vi "STORE_INPUT.vi"(9 "CURRENT_YEAR_DATA":string, 10 "connection reference":T1, 11 "ECODE 2":string) -> ()   [LabVIEW 2015]
uses:
  <vilib>/addons/database/Connection.llb/Conn ObjectReference.ctl
  <vilib>/Utility/miscctls.llb/LVRowAndColumnUnsignedTypeDef.ctl
  Controls/STORE_INPUT_NO_CLUSTER.ctl
  Controls/STORE_INPUT_INFORMATION_Cluster.ctl
  Controls/ITEM_INFORMATION_CLUSTER.ctl
  Controls/Print_Data.ctl
  <vilib>/addons/database/Connection.llb/Conn Execute.vi
  <vilib>/addons/database/Recordset.llb/Rec Destroy - Connection.vi
  <vilib>/addons/database/_DB Variant To Data/Database Variant To Data.xnode
  <vilib>/addons/database/NI_Database_API.lvlib
  <vilib>/addons/database/Connection.llb/DB Tools Open Connec (String).vi
panel:
  in  "AUTO_PRINT":bool caption="AUTO"
  in  "PRINT button":bool
  in  "Lot Maker":string
  in  "Next Button":bool
  out "Find Array":i32[](array[numeric])
  in  "Location":string
  in  "Maker Code":string
  in  "Excle Path (F1)":path
  in  "BUTTON_EXIT":bool
  in  "BUTTON_INPUT":bool
  in  "BUTTON_ADD":bool
  in  "Search":string
  in  "Amount (F4)":dbl caption="(F4)"
  in  "Unit 2":string
  in  "Quantity":dbl
  in  "Lot Size":dbl
  in  "Unit":string
  in  "Item Code (F3)":string
  in  "Part No (F2)":string
  in  "Barcode (F1)":string
  in  "Offset":dbl
  in  "Length":dbl
  in  "Maker":string(combo)
  in  "Part Name":string(combo)
  in  "Product":string(combo)
  out "ECODE":string
  in  "Input Date":timestamp format="%<%d/%m/%Y>T"
  out "Input No.":string
  out "Table":string[][](table)
  # "INPUT"
  # "X"
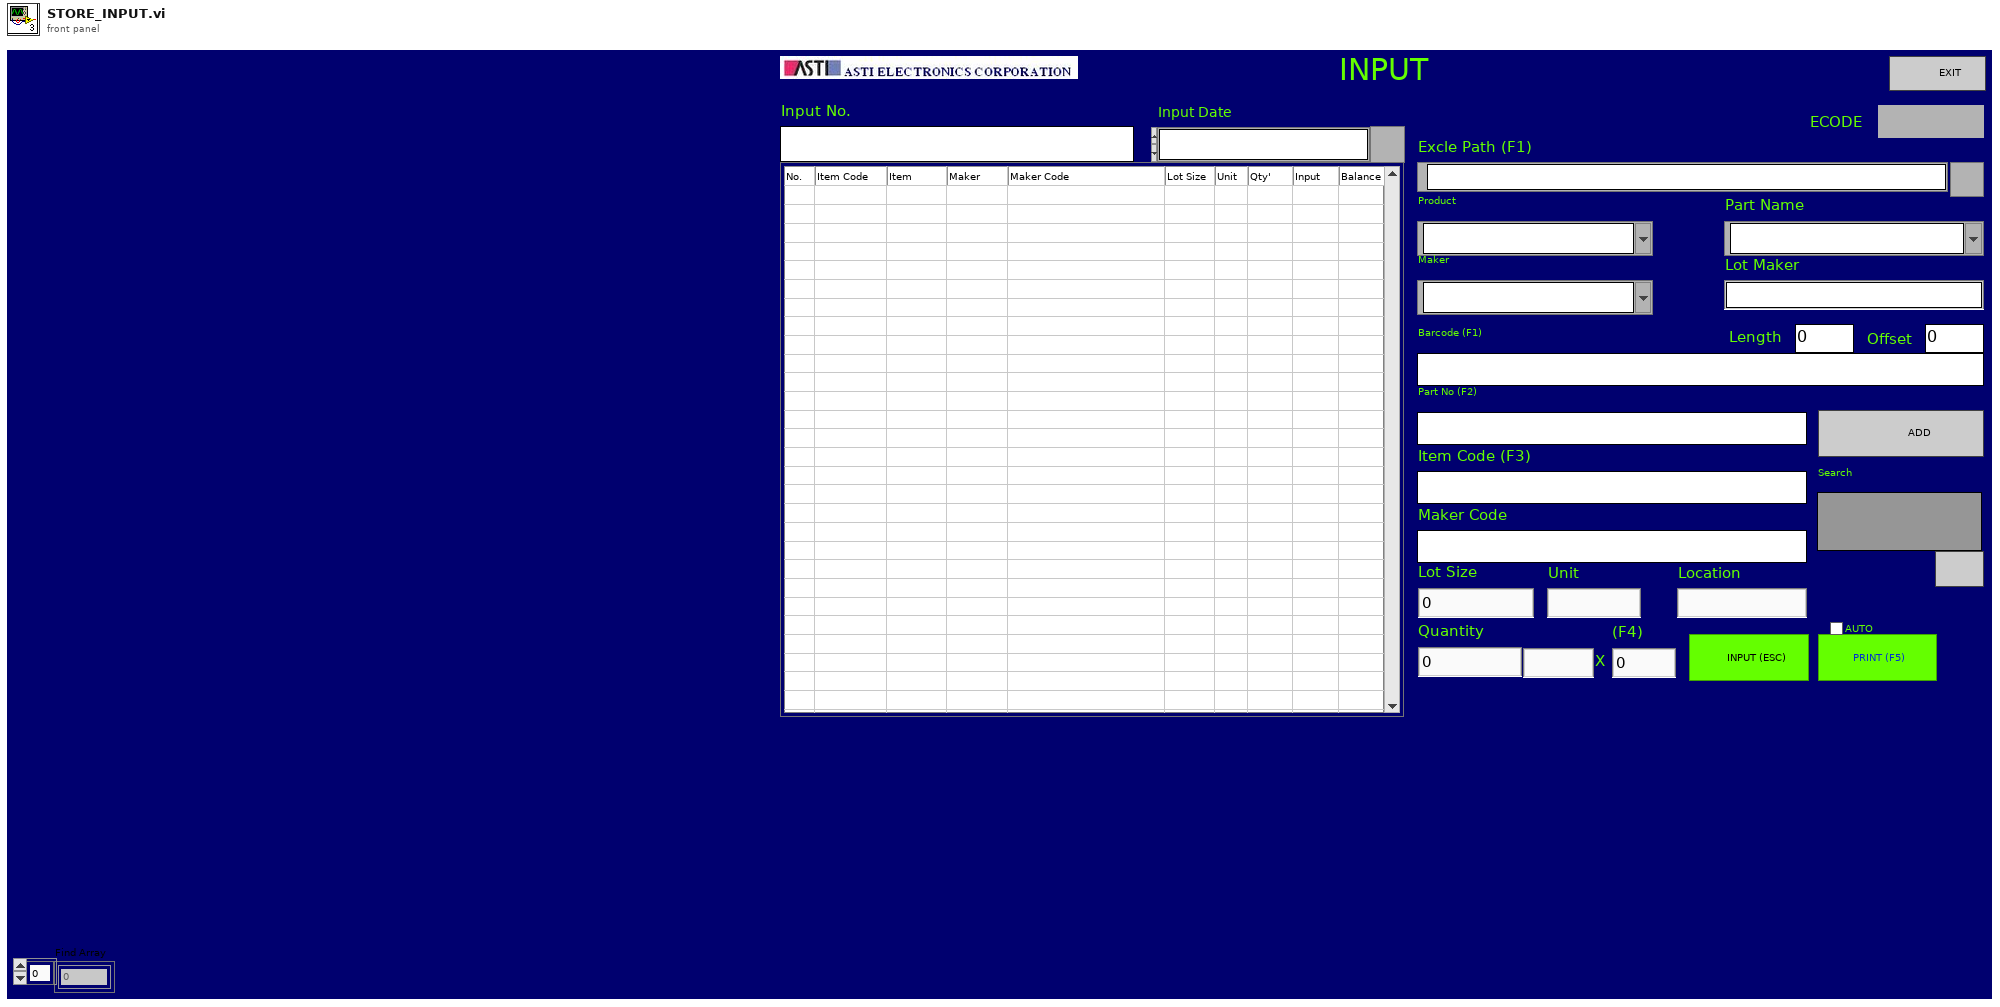
[diagram p1: front panel]
types:
  T1 = typedef "NI_Database_API.lvlib/Conn ObjectReference.ctl" = refnum<k1>
  T2 = typedef "LVRowAndColumnUnsignedTypeDef.ctl" = cluster{"Row":u32, "Column":u32}
  T3 = typedef "STORE_INPUT_NO_CLUSTER.ctl" = cluster{"NO":dbl, "ITEM_CODE":string, "ITEM":string, "MAKER":string, "MAKER_CODE":string, "LOT_SIZE":dbl, "UNIT":string, "QUANTITY":dbl, "INPUT":dbl, "BALANCE":dbl, "DESTINATION":string, "INVOICE_NO":string}
  T4 = cluster{"start (-1, -1)":cluster{"row":i32, "column":i32}, "end (-1, -1)":cluster{"row":i32, "column":i32}}
  T5 = typedef "STORE_INPUT_INFORMATION_Cluster.ctl" = cluster{"INPUT_NO":string, "INPUT_DATE":timestamp, "ECODE":string}
  T6 = typedef "ITEM_INFORMATION_CLUSTER.ctl" = cluster{"PRODUCT":string, "ITEM_CODE":string, "PART_NAME":string, "MAKER":string, "PART_NO":string, "LOT_SIZE":dbl, "UNIT":string, "LENGTH-OFFSET":string, "BARCODE":string, "PROCESS":string, "INVENTORY_LOCAL":string, "TARE":dbl, "SAMPLE":dbl}
  T7 = typedef "Print_Data.ctl" = cluster{"QR_code Text":string, "Lot Maker":string, "Item Code (F3)":string, "date/time string":string, "Invoice No.":string, "Maker":string, "Part No.(F2) ":string, "Location":string, "Product":string, "Qty":string, "ECODE":string}
  T8 = cluster{"ITEM_CODE":string, "INVOICE_NO":string, "INVOICE_DATE":timestamp, "LOT_MAKER":string, "QUANTITY":dbl, "INVOICE_ECODE":string, "INPUT_NO":string, "INPUT_DATE":timestamp, "INPUT_ECODE":string, "LINEBACK_NO":string, "LINEBACK_DATE":timestamp, "LINEBACK_ECODE":string, "OUTPUT_NO":string, "OUTPUT_DATE":timestamp, "OUTPUT_ECODE":string, "DESTINATION":string}
  T9 = cluster{"PRODUCT":string, "ITEM CODE":string, "PART NAME":string, "MAKER":string, "PART NO":string, "LOT SIZE":dbl, "UNIT":string, "LENGTH-OFFSET":string, "BARCODE":string, "PROCESS":string, "INVENTORY LOCAL":string, "TARE":dbl, "SAMPLE":dbl}
  T10 = typedef "NI_Database_API.lvlib/Rec ObjectReference.ctl" = refnum<k1>
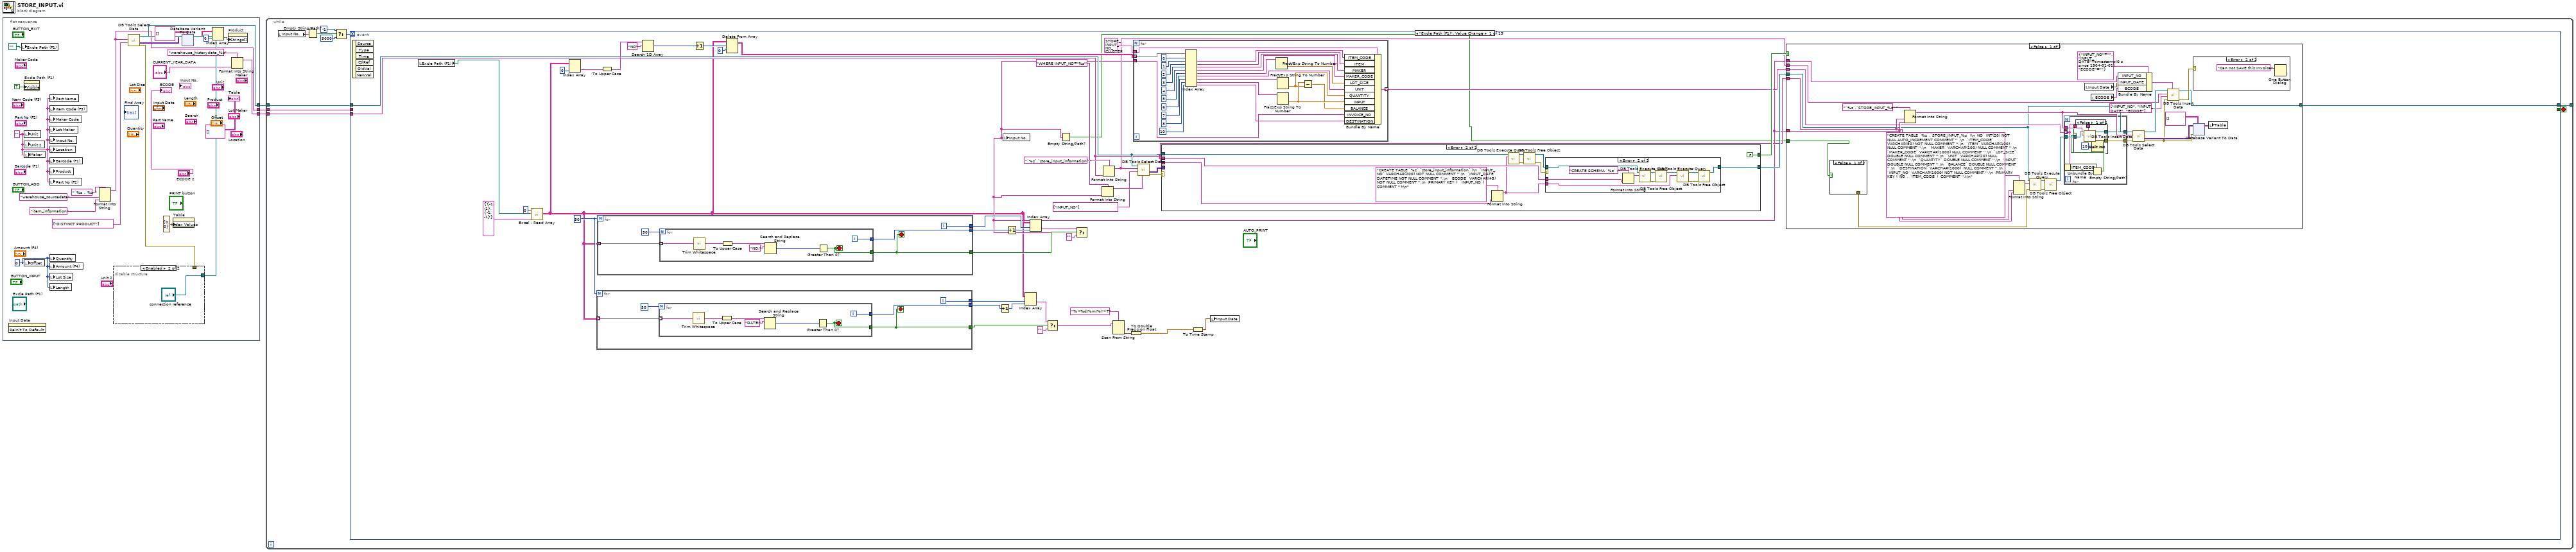
[diagram p0: block diagram]
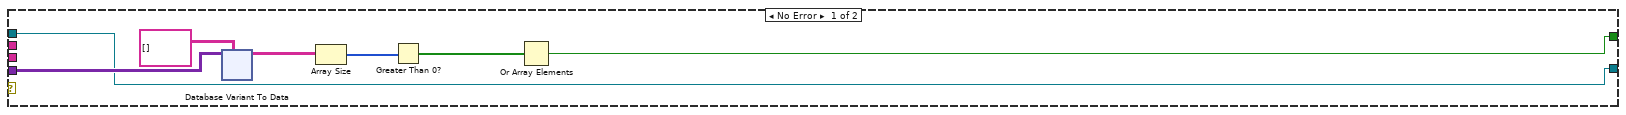
[diagram p2: hidden frame]
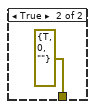
[diagram p4: hidden frame]
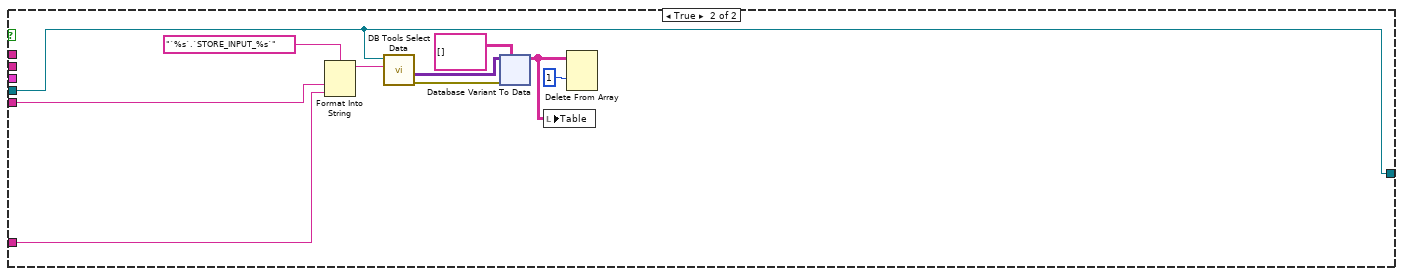
[diagram p7: hidden frame]
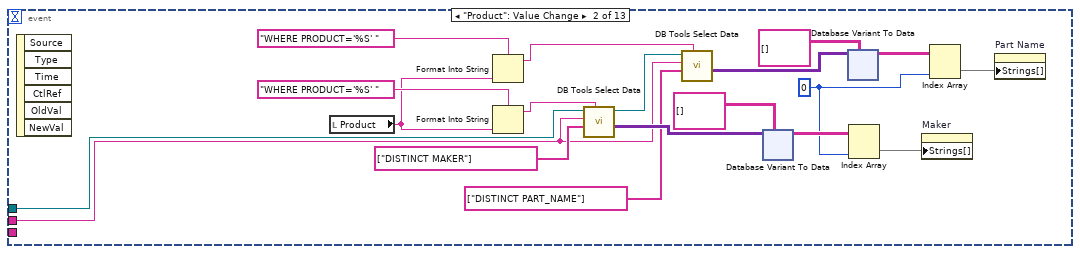
[diagram p8: hidden frame]
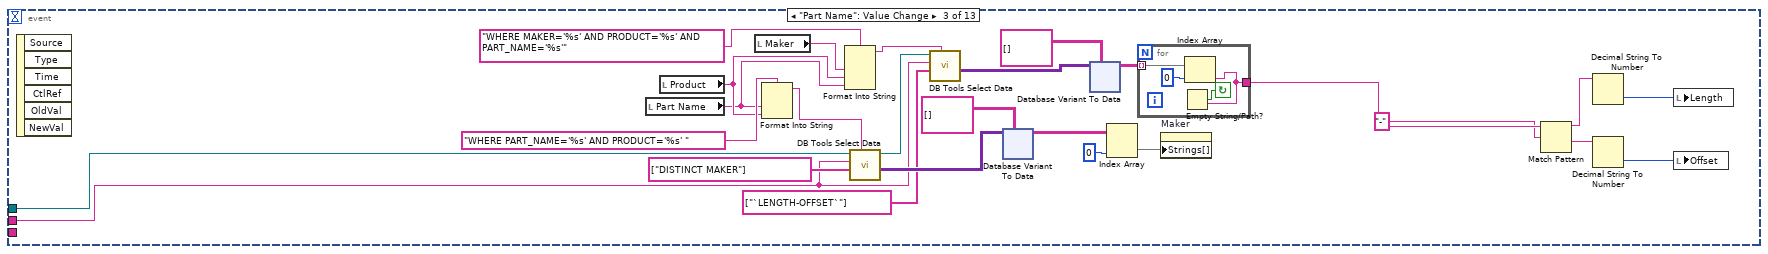
[diagram p9: hidden frame]
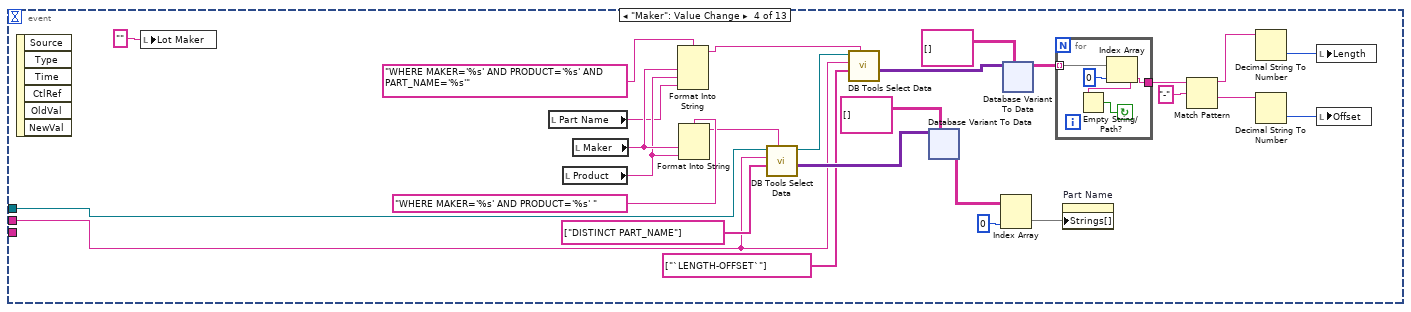
[diagram p10: hidden frame]
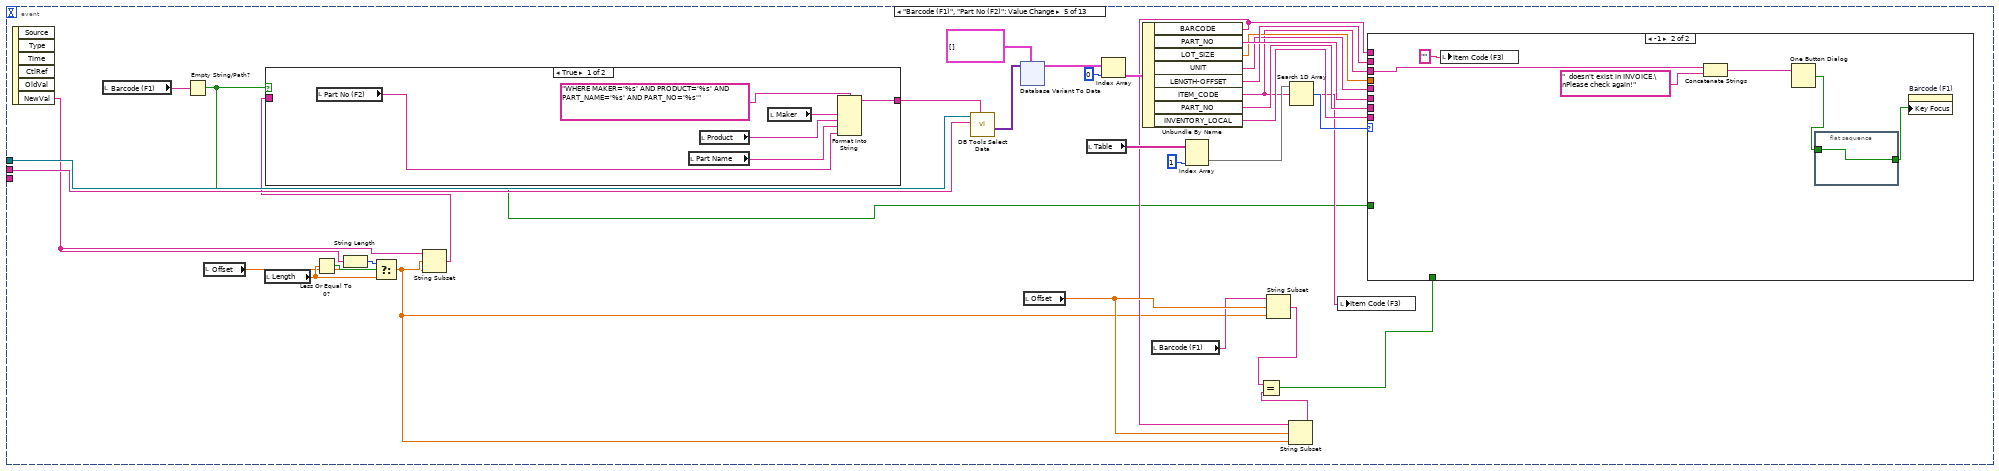
[diagram p11: hidden frame]
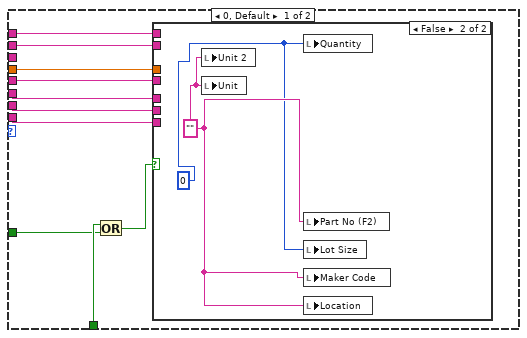
[diagram p12: hidden frame]
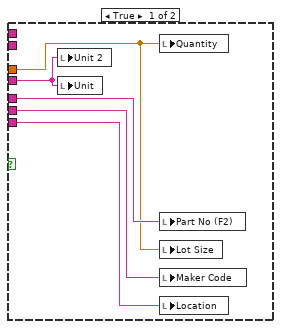
[diagram p13: hidden frame]
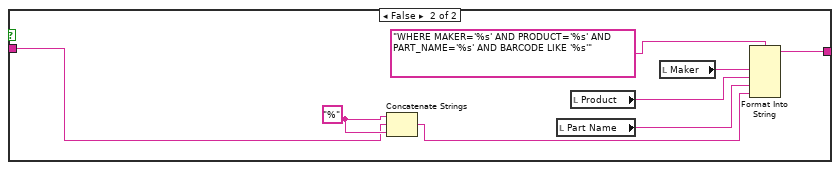
[diagram p14: hidden frame]
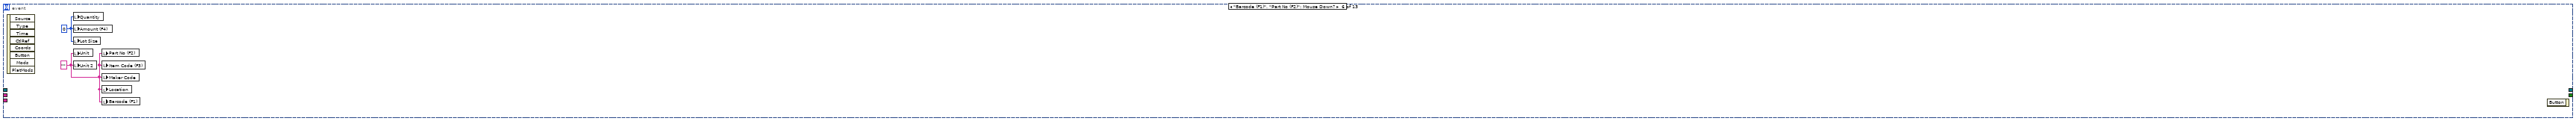
[diagram p15: hidden frame]
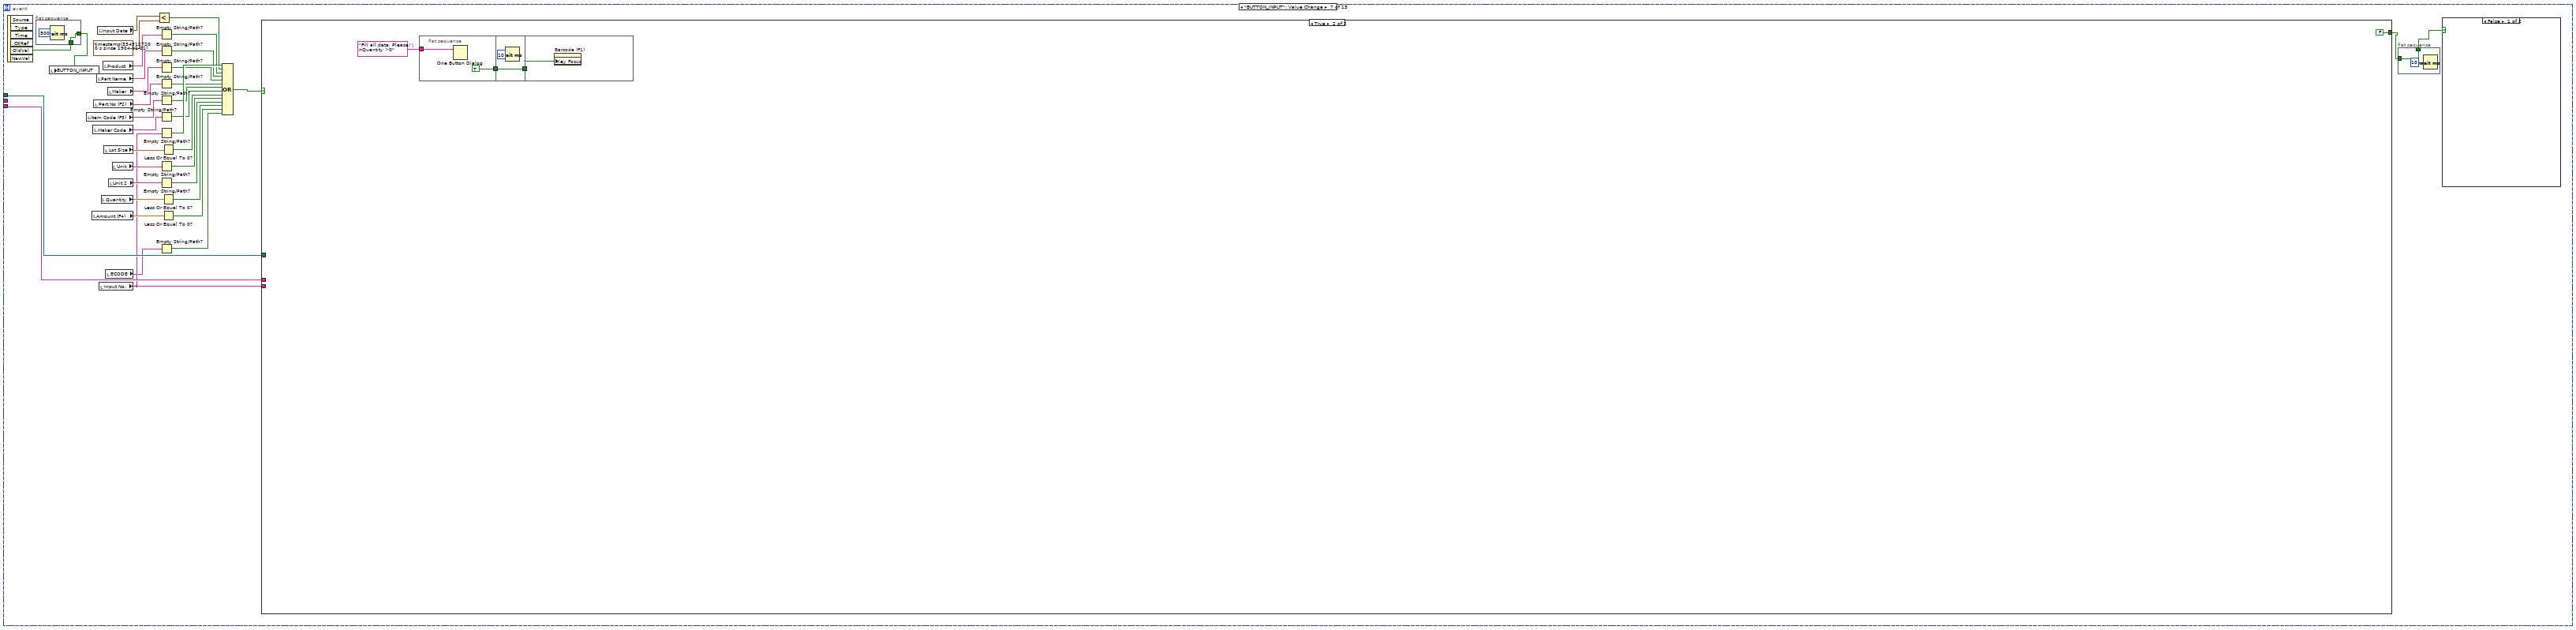
[diagram p16: hidden frame]
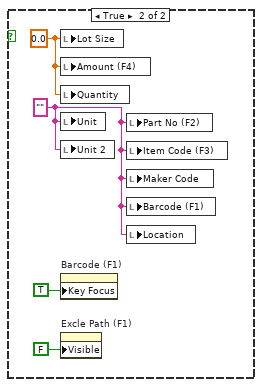
[diagram p17: hidden frame]
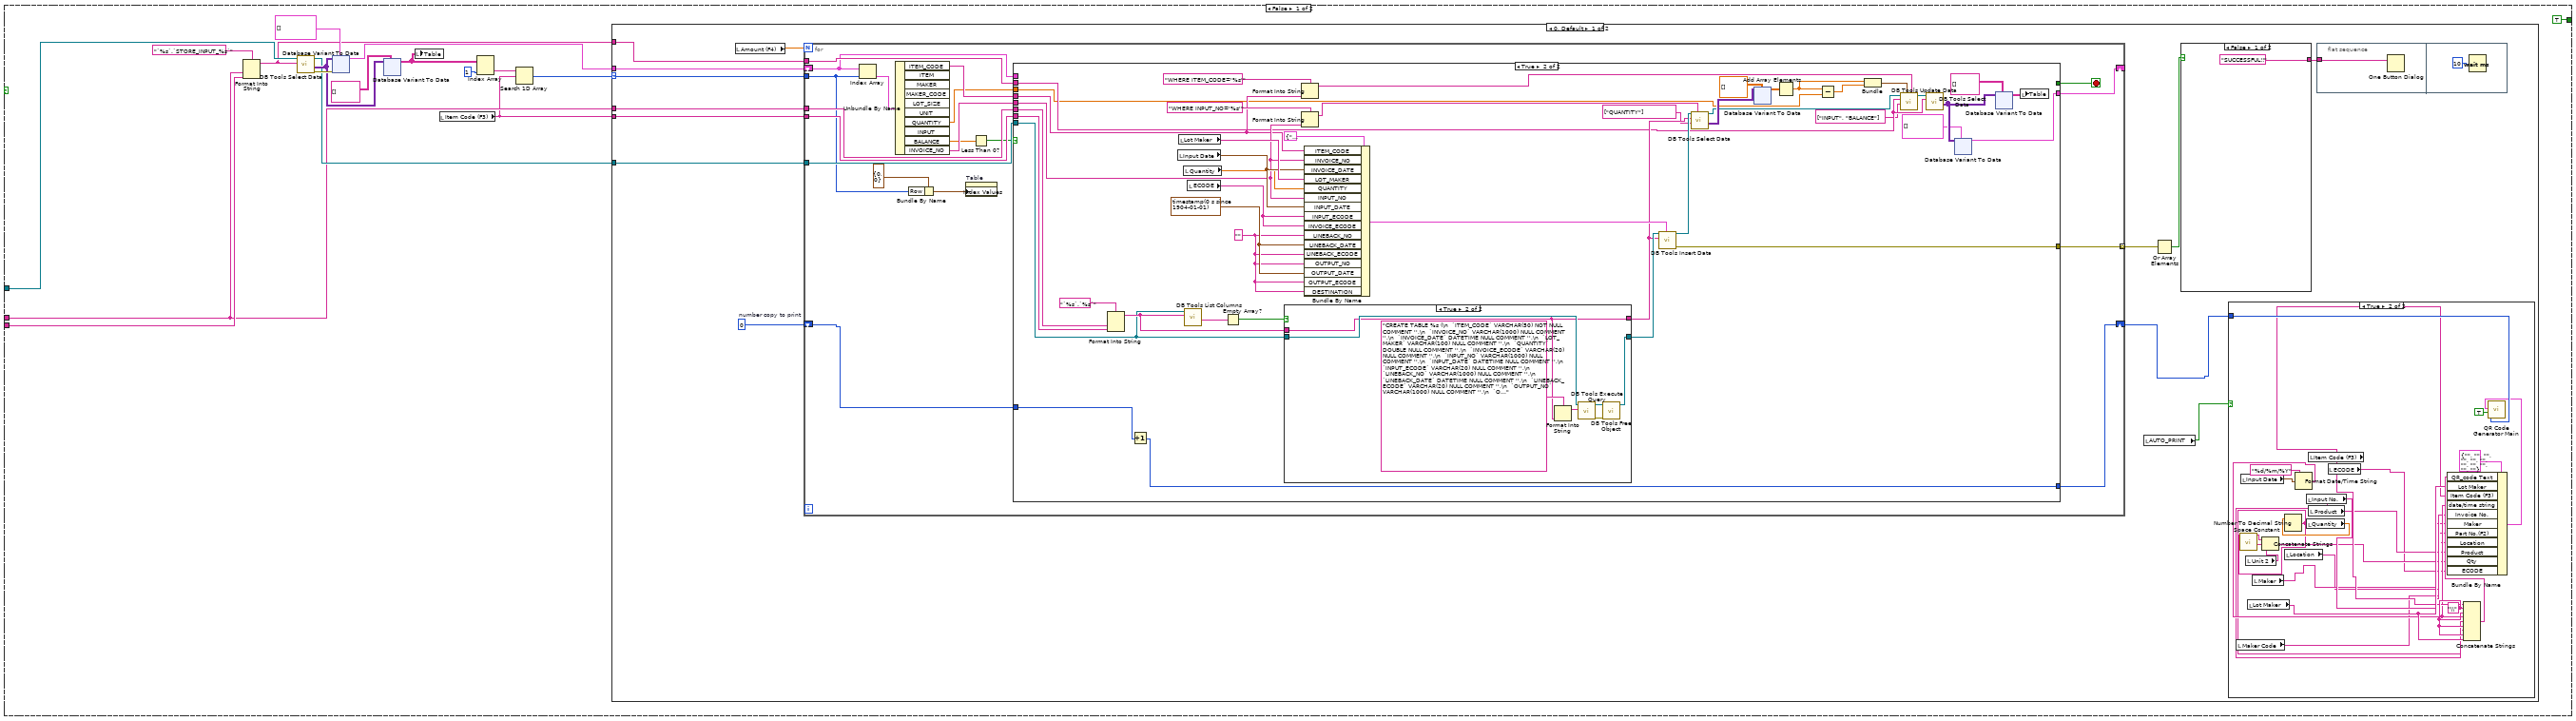
[diagram p18: hidden frame]
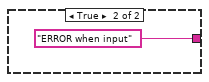
[diagram p20: hidden frame]
diagram:
  n1 = flat-sequence {
    tunnel: [w22] -> w3
    tunnel: [w16] -> w2
    tunnel: [w12] -> w1
    frame #0 {
      w10 = 0
      w8 = ""
      n2 = invoke on="Input Date" class="AbsTime (strict)" method="Reinit To Default"() -> ()  [unwired: 3 in, 3 out]
      n3 = local write "Excle Path (F1)"(path "" ("Excle Path")) -> ()
      n4 = property on="Excle Path (F1)" class="Path"("Visible"=TRUE) -> ()  [unwired: 2 in, 2 out]
      n5 = local write "Unit"(w8) -> ()
      n6 = local write "Unit 2"(w8) -> ()
      n7 = local write "Maker"(w8) -> ()
      n8 = local write "Offset"(w10) -> ()
      n9 = local write "Part Name"(w8) -> ()
      n10 = local write "Item Code (F3)"(w8) -> ()
      n11 = local write "Maker Code"(w8) -> ()
      n12 = local write "Lot Maker"(w8) -> ()
      n13 = local write "Input No."(w8) -> ()
      n14 = local write "Location"(w8) -> ()
      n15 = local write "Barcode (F1)"(w8) -> ()
      n16 = local write "Product"(w8) -> ()
      n17 = local write "Part No (F2)"(w8) -> ()
      n18 = local write "Quantity"(w10) -> ()
      n19 = local write "Amount (F4)"(w10) -> ()
      n20 = local write "Lot Size"(w10) -> ()
      n21 = local write "Length"(w10) -> ()
      n22 = Format Into String(format string="`%s`.`%s`" ("table"), "warehouse_sourcedata" ("table"), "item_information" ("table")) -> (resulting string=w16:string)  [unwired: 2 in, 1 out]
      n23 = disable-structure shown="Enabled" {
        disable-tunnel: [w28 "connection reference"] -> w24
        disable-tunnel: [w27 _] -> w23
        frame Disabled {
          n24 = call-poly <vilib>:"DB Tools Open Connection.vi"("password"="871994" ("userID"), "userID"="hoangbao2106", "connection information"="Database" ("userID")) -> ("error out"=w27:errorcluster, "connection reference"=w28:T1)  [unwired: 5 in]
        }
        frame Enabled {
        }
      }
      n25 = call <vilib>:"DB Tools Select Data.vi"("error in (no error)"=w23, "columns"=string[] ["DISTINCT PRODUCT"], "table"=w16, "connection reference"=w24) -> ("data"=w21:variant[][], "connection reference out"=w22:T1)  [unwired: 2 in, 1 out]
      n26 = property on="Table" class="Tbl (strict)"("Index Values"=T2 {"Row"=0, "Column"=0}) -> ()  [unwired: 2 in, 2 out]
      n27 = xnode "Database Variant To Data"("database variant"=w21, "type"=string[][] []) -> ("data"=w18:string[][])  [unwired: 1 in, 1 out]
      n28 = Index Array(array=w18, index (col)=0 ("index (row)")) -> (element=w17:string[])  [unwired: 1 in]
      n29 = property on="Product" class="CmbBox"("Strings[]"=w17) -> ()  [unwired: 2 in, 2 out]
      n30 = Format Into String(format string="warehouse_historydata_%s" ("table"), "CURRENT_YEAR_DATA") -> (resulting string=w12:string)  [unwired: 2 in, 1 out]
      "Table" <- string[][] [] ("Table")
      "ECODE" <- "ECODE 2"
    }
  }
  n31 = while {
    tunnel: w3 -> [w85]
    tunnel: w2 -> [w84]
    tunnel: w1 -> [w83]
    tunnel: [w82] -> _
    stop <- w86 stop-if-true
    n32 = local read "Input No."() -> (w81:string)
    n33 = Empty String/Path?(string/path=w81) -> (empty?=w80:bool)
    n34 = Select(t=-1, s=w80, f=5000) -> (s? t:f=w78:i32)
    n35 = event shown="[0] \"Excle Path (F1)\": Value Change" {
      selector: _ -> [_ _ _ _ _ _ _ _ _ _ _ _ _]
      dyn-events: _ -> [_ _ _ _ _ _ _ _ _ _ _ _ _]
      timeout: w78 -> [_ _ _ _ _ _ _ _ _ _ _ _ _]
      tunnel: [_ _ _ _ _ _ _ _ _ _ _ _ TRUE] -> w86
      tunnel: w85 -> [w110 w414 w525 w644 w775 _ w1239 _ w2362 w2395 _ _ _]
      tunnel: w84 -> [_ w401 w510 w640 w774 _ _ _ _ _ _ _ _]
      tunnel: w83 -> [w108 _ _ _ _ _ w1238 _ _ w2394 _ _ _]
      tunnel: [w103 _ _ _ _ _ _ _ _ _ _ _ _] -> w82
      event "Excle Path (F1)": Value Change {
        w100 = 50
        n36 = event-data() -> ()  [unwired: 1 in, 6 out]
        n37 = local read "Excle Path (F1)"() -> (w132:path)
        n38 = call "Excel - Read Array.vi"("Cluster"=T4 {"start (-1, -1)"={"row"=-1, "column"=-1}, "end (-1, -1)"={"row"=-1, "column"=-1}}, "Path"=w132, "worksheet index (0)"=0) -> ("Element 1"=w99:string[][])  [unwired: 5 in, 1 out]
        n39 = Index Array(array=w99, index (col)=0 ("disabled index (col)")) -> (element=w122:string[])  [unwired: 1 in]
        n40 = for {
          N: w100 -> [_]
          tunnel: w99 -> [w137] mode=indexing
          tunnel: [w136] -> w98
          tunnel: [w134] -> w97
          tunnel: [w133] -> w94
          i -> [w136]
          stop <- w133 stop-if-true
          n41 = for {
            N: 50 -> [_]
            tunnel: w137 -> [w143] mode=indexing
            tunnel: [w138] -> w133
            tunnel: [w144] -> w134
            i -> [w144]
            stop <- w138 stop-if-true
            n42 = call <vilib>:"Trim Whitespace.vi"("string"=w143) -> ("trimmed string"=w142:string)  [unwired: 1 in]
            n43 = To Upper Case(1:w142) -> (0:w141:string)
            n44 = Search and Replace String(input string=w141, search string="DATE:" ("y")) -> (number of replacements=w139:i32)  [unwired: 6 in, 3 out]
            n45 = Greater Than 0?(x=w139) -> (x > 0?=w138:bool)
          }
        }
        n46 = for {
          N: w100 -> [_]
          tunnel: w99 -> [w392] mode=indexing
          tunnel: [w391] -> w127
          tunnel: [w389] -> w129
          tunnel: [w388] -> w130
          i -> [w391]
          stop <- w388 stop-if-true
          n47 = for {
            N: 50 -> [_]
            tunnel: w392 -> [w398] mode=indexing
            tunnel: [w393] -> w388
            tunnel: [w399] -> w389
            i -> [w399]
            stop <- w393 stop-if-true
            n48 = call <vilib>:"Trim Whitespace.vi"("string"=w398) -> ("trimmed string"=w397:string)  [unwired: 1 in]
            n49 = To Upper Case(1:w397) -> (0:w396:string)
            n50 = Search and Replace String(input string=w396, search string="NO:" ("y")) -> (number of replacements=w394:i32)  [unwired: 6 in, 3 out]
            n51 = Greater Than 0?(x=w394) -> (x > 0?=w393:bool)
          }
        }
        n52 = To Upper Case(1:w122) -> (0:w121:string[])
        n53 = Search 1D Array(1D array=w121, element="NO") -> (index of element=w120:i32)  [unwired: 1 in]
        n54 = Increment(x=w120) -> (x+1=w119:i32)
        n55 = Delete From Array(array=w99, length=w119, index (row)=0) -> (array with subset deleted=w107:string[][])  [unwired: 1 in, 1 out]
        n56 = Increment(x=w97) -> (x+1=w96:i32)
        n57 = Increment(x=w129) -> (x+1=w128:i32)
        n58 = Index Array(array=w99, index (row)=w98, index (col)=w96) -> (element=w93:string)
        n59 = Index Array(array=w99, index (row)=w127, index (col)=w128) -> (element=w126:string)
        n60 = Select(t=w93, s=w94, f="") -> (s? t:f=w90:string)
        n61 = Select(t=w126, s=w130, f="") -> (s? t:f=w102:string)
        n62 = local write "Input No."(w102) -> ()
        n63 = Empty String/Path?(string/path=w102) -> (empty?=w101:bool)
        n64 = Format Into String(format string="WHERE INPUT_NO='%s'", w102) -> (resulting string=w115:string)  [unwired: 2 in, 1 out]
        n65 = Format Into String(format string="`%s`.`store_input_information` ", w108) -> (resulting string=w104:string)  [unwired: 2 in, 1 out]
        n66 = Scan From String(format string="%<%d/%m/%Y>T", input string=w90) -> (output 1=w91:timestamp)  [unwired: 3 in, 3 out]
        n67 = To Double Precision Float(number=w91) -> (double precision float=w89:dbl)
        n68 = for {
          tunnel: w107 -> [w170] mode=indexing
          tunnel: T3 {"NO"=0.0, "ITEM_CODE"="", "ITEM"="", "MAKER"="", "MAKER_CODE"="", "LOT_SIZE"=0.0, "UNIT"="", "QUANTITY"=0.0, "INPUT"=0.0, "BALANCE"=0.0, "DESTINATION"="", "INVOICE_NO"=""} -> [w171]
          tunnel: [w150] -> w105 mode=indexing
          tunnel: w102 -> [w149]
          n69 = Index Array(array=w170, index #1=0 ("index"), index #2=1 ("index"), index #3=2 ("index"), index #4=3 ("index"), index #5=4 ("index"), index #6=5 ("index"), index #7=6 ("index"), index #8=7 ("index"), index #9=8 ("index"), index #10=10 ("index")) -> (element #2=w159:string, element #3=w158:string, element #4=w157:string, element #5=w156:string, element #6=w155:string, element #7=w153:string, element #8=w152:string, element #9=w151:string, element #10=w145:string)  [unwired: 1 out]
          n70 = Fract/Exp String To Number(string=w155) -> (number=w154:dbl)  [unwired: 3 in, 1 out]
          n71 = Fract/Exp String To Number(string=w152) -> (number=w147:dbl)  [unwired: 3 in, 1 out]
          n72 = Fract/Exp String To Number(string=w151) -> (number=w148:dbl)  [unwired: 3 in, 1 out]
          n73 = Subtract(x=w148, y=w147) -> (x-y=w146:dbl)
          n74 = Bundle By Name(cluster=w171, "ITEM_CODE"=w159, "ITEM"=w158, "MAKER"=w157, "MAKER_CODE"=w156, "LOT_SIZE"=w154, "UNIT"=w153, "QUANTITY"=w147, "INPUT"=w148, "BALANCE"=w146, "INVOICE_NO"=w149, "DESTINATION"=w145) -> (w150:T3)
        }
        n75 = call <vilib>:"DB Tools Select Data.vi"("condition"=w115, "columns"=string[] ["INPUT_NO"], "table"=w104, "connection reference"=w110) -> ("error out"=w111:errorcluster, "data"=w114:variant[][])  [unwired: 2 in, 1 out]
        n76 = case shown="Error" w111 {
          tunnel: w114 -> [w178 _]
          tunnel: [w173 FALSE] -> w112
          tunnel: w110 -> [w172 w230]
          tunnel: [w172 w226] -> w109
          tunnel: w108 -> [_ w228]
          tunnel: w108 -> [_ w224]
          frame No Error {
            n77 = xnode "Database Variant To Data"("database variant"=w178, "type"=string[][] []) -> ("data"=w176:string[][])  [unwired: 1 in, 1 out]
            n78 = Array Size(array=w176) -> (size(s)=w175:i32[])
            n79 = Greater Than 0?(x=w175) -> (x > 0?=w174:bool[])
            n80 = Or Array Elements(Boolean array=w174) -> (logical OR=w173:bool)
          }
          frame Error {
            n81 = Format Into String(format string="CREATE TABLE `%s`.`store_input_information` (\n  `INPUT_NO` VARCHAR(200) NOT NULL COMMENT '',\n  `INPUT_DATE` DATETIME NOT NULL COMMENT '',\n  `ECODE` VARCHAR(45) NOT NULL COMMENT '',\n  PRIMARY KEY (  `INPUT_NO`)  COMMENT '');\n", w224) -> (resulting string=w223:string)  [unwired: 2 in, 1 out]
            n82 = call-poly <vilib>:"DB Tools Execute Query.vi"("SQL query"=w223, "connection reference"=w230) -> ("error out"=w232:errorcluster, "recordset reference"=w233:T10)  [unwired: 6 in]
            n83 = call-poly <vilib>:"DB Tools Free Object.vi"("error in (no error)"=w232, "recordset reference"=w233) -> ("error out"=w229:errorcluster, "connection reference"=w227:T1)  [unwired: 8 in]
            n84 = case shown="Error" w229 {
              tunnel: w227 -> [w234 w245]
              tunnel: w228 -> [_ w243]
              tunnel: w223 -> [_ w237]
              tunnel: [w234 w236] -> w226
              frame No Error {
              }
              frame Error {
                n85 = Format Into String(format string="CREATE SCHEMA `%s` ;" ("SQL query"), w243) -> (resulting string=w235:string)  [unwired: 2 in, 1 out]
                n86 = call-poly <vilib>:"DB Tools Execute Query.vi"("SQL query"=w235, "connection reference"=w245) -> ("error out"=w241:errorcluster, "recordset reference"=w242:T10)  [unwired: 6 in]
                n87 = call-poly <vilib>:"DB Tools Free Object.vi"("error in (no error)"=w241, "recordset reference"=w242) -> ("connection reference"=w238:T1)  [unwired: 8 in, 1 out]
                n88 = call-poly <vilib>:"DB Tools Execute Query.vi"("SQL query"=w237, "connection reference"=w238) -> ("error out"=w240:errorcluster, "recordset reference"=w239:T10)  [unwired: 6 in]
                n89 = call-poly <vilib>:"DB Tools Free Object.vi"("error in (no error)"=w240, "recordset reference"=w239) -> ("connection reference"=w236:T1)  [unwired: 8 in, 1 out]
              }
            }
          }
        }
        n90 = To Time Stamp(1:w89) -> (0:w88:timestamp)
        n91 = local write "Input Date"(w88) -> ()
        n92 = case shown="False" w112 {
          tunnel: w109 -> [w246 w343]
          tunnel: w108 -> [w269 w337]
          tunnel: w102 -> [w268 w338]
          tunnel: [w255 w343] -> w103
          tunnel: w105 -> [w267 _]
          tunnel: w104 -> [w258 _]
          tunnel: w102 -> [w254 _]
          tunnel: w101 -> [w248 _]
          frame False {
            n93 = case shown="False" w248 {
              tunnel: [_ errorcluster {"status"=TRUE, "code"=0, "source"=""} ("error constant")] -> w247
              frame False {
              }
              frame True {
              }
            }
            n94 = Format Into String(format string="`%s`.`STORE_INPUT_%s` " ("SQL query"), w269, w268) -> (resulting string=w262:string)  [unwired: 2 in, 1 out]
            n95 = Format Into String(format string="CREATE TABLE `%s`.`STORE_INPUT_%s` (\n`NO` INT(20) NOT NULL AUTO_INCREMENT COMMENT '' ,\n  `ITEM_CODE` VARCHAR(50) NOT NULL COMMENT '',\n  `ITEM` VARCHAR(100) NULL COMMENT '',\n  `MAKER` VARCHAR(100) NULL COMMENT '',\n  `MAKER_CODE` VARCHAR(1000) NULL COMMENT '',\n  `LOT_SIZE` DOUBLE NULL COMMENT '',\n  `UNIT` VARCHAR(20) NULL COMMENT '',\n  `QUANTITY` DOUBLE NULL COMMENT '',\n  `INPUT` DOUBLE NULL COMMENT '',\n  `BALANCE` DOUBLE NULL COMMENT '',\n  `DESTINATION` VARCHAR(1000)  NULL COMMENT '',\n  `INPUT_NO` VARCHAR(1000) NOT NULL COMMENT '',\n  PRIMARY KEY (`NO`, `ITEM_CODE`)  COMMENT '');\n" ("SQL query"), w269, w268) -> (resulting string=w261:string)  [unwired: 2 in, 1 out]
            n96 = call-poly <vilib>:"DB Tools Execute Query.vi"("error in (no error)"=w247, "SQL query"=w261, "connection reference"=w246) -> ("error out"=w271:errorcluster, "recordset reference"=w272:T10)  [unwired: 5 in]
            n97 = call-poly <vilib>:"DB Tools Free Object.vi"("error in (no error)"=w271, "recordset reference"=w272) -> ("connection reference"=w263:T1)  [unwired: 8 in, 1 out]
            n98 = for {
              tunnel: w263 -> [w326]
              tunnel: w262 -> [w325]
              tunnel: w267 -> [w322] mode=indexing
              tunnel: [w324] -> _
              tunnel: [w323] -> w260
              n99 = Unbundle By Name(w322) -> ("ITEM_CODE"=w321:string)
              n100 = Empty String/Path?(string/path=w321) -> (empty?=w320:bool)
              n101 = case shown="False" w320 {
                tunnel: w326 -> [w332 w333]
                tunnel: w325 -> [w331 _]
                tunnel: w322 -> [w330 _]
                tunnel: [w329 w333] -> w324
                tunnel: [w328 _] -> w323
                frame False {
                  n102 = call <vilib>:"DB Tools Insert Data.vi"("data"=w330, "table"=w331, "connection reference"=w332) -> ("error out"=w328:errorcluster, "connection reference out"=w329:T1)  [unwired: 7 in]
                  n103 = Wait (ms)(milliseconds to wait=u32 10) -> ()  [unwired: 1 out]
                }
                frame True {
                }
              }
            }
            n104 = local read "Input Date"() -> (w253:timestamp)
            n105 = local read "ECODE"() -> (w252:string)
            n106 = Bundle By Name(cluster=T5 {"INPUT_NO"="", "INPUT_DATE"=timestamp(0 s since 1904-01-01), "ECODE"=""} ("INVOICE_INFORMATION_Cluster"), "INPUT_NO"=w254, "INPUT_DATE"=w253, "ECODE"=w252) -> (w251:T5)
            n107 = call <vilib>:"DB Tools Select Data.vi"("error in (no error)"=w260, "table"=w262, "connection reference"=w246) -> ("error out"=w257:errorcluster, "data"=w266:variant[][], "connection reference out"=w259:T1)  [unwired: 3 in]
            n108 = call <vilib>:"DB Tools Insert Data.vi"("data"=w251, "error in (no error)"=w257, "columns"=string[] ["INPUT_NO", "INPUT_DATE", "ECODE"], "table"=w258, "connection reference"=w259) -> ("error out"=w256:errorcluster, "connection reference out"=w255:T1)  [unwired: 5 in]
            n109 = case shown="Error" w256 {
              frame No Error {
              }
              frame Error {
                n110 = One Button Dialog(message="Can not SAVE this Invoice") -> ()  [unwired: 1 in, 1 out]
              }
            }
            n111 = xnode "Database Variant To Data"("database variant"=w266, "error in (no error)"=w257, "type"=string[][] []) -> ("data"=w264:string[][])  [unwired: 1 out]
            n112 = local write "Table"(w264) -> ()
          }
          frame True {
            n113 = Format Into String(format string="`%s`.`STORE_INPUT_%s`", w337, w338) -> (resulting string=w336:string)  [unwired: 2 in, 1 out]
            n114 = call <vilib>:"DB Tools Select Data.vi"("table"=w336, "connection reference"=w343) -> ("error out"=w340:errorcluster, "data"=w342:variant[][])  [unwired: 4 in, 1 out]
            n115 = xnode "Database Variant To Data"("database variant"=w342, "error in (no error)"=w340, "type"=string[][] []) -> ("data"=w335:string[][])  [unwired: 1 out]
            n116 = local write "Table"(w335) -> ()
            n117 = Delete From Array(array=w335, index (row)=1) -> ()  [unwired: 2 in, 2 out]
          }
        }
      }
      event "Product": Value Change {
        w400 = 0 ("index (row)")
        n118 = event-data() -> ()  [unwired: 1 in, 6 out]
        n119 = local read "Product"() -> (w405:string)
        n120 = Format Into String(format string="WHERE PRODUCT='%S' " ("condition"), w405) -> (resulting string=w411:string)  [unwired: 2 in, 1 out]
        n121 = Format Into String(format string="WHERE PRODUCT='%S' " ("condition"), w405) -> (resulting string=w412:string)  [unwired: 2 in, 1 out]
        n122 = call <vilib>:"DB Tools Select Data.vi"("condition"=w412, "columns"=string[] ["DISTINCT MAKER"], "table"=w401, "connection reference"=w414) -> ("data"=w415:variant[][], "connection reference out"=w404:T1)  [unwired: 2 in, 1 out]
        n123 = call <vilib>:"DB Tools Select Data.vi"("condition"=w411, "columns"=string[] ["DISTINCT PART_NAME"], "table"=w401, "connection reference"=w404) -> ("data"=w409:variant[][])  [unwired: 2 in, 2 out]
        n124 = xnode "Database Variant To Data"("database variant"=w415, "type"=string[][] []) -> ("data"=w418:string[][])  [unwired: 1 in, 1 out]
        n125 = xnode "Database Variant To Data"("database variant"=w409, "type"=string[][] []) -> ("data"=w406:string[][])  [unwired: 1 in, 1 out]
        n126 = Index Array(array=w418, index (col)=w400) -> (element=w402:string[])  [unwired: 1 in]
        n127 = property on="Maker" class="CmbBox"("Strings[]"=w402) -> ()  [unwired: 2 in, 2 out]
        n128 = Index Array(array=w406, index (col)=w400) -> (element=w403:string[])  [unwired: 1 in]
        n129 = property on="Part Name" class="CmbBox"("Strings[]"=w403) -> ()  [unwired: 2 in, 2 out]
      }
      event "Part Name": Value Change {
        n130 = event-data() -> ()  [unwired: 1 in, 6 out]
        n131 = local read "Part Name"() -> (w507:string)
        n132 = local read "Product"() -> (w508:string)
        n133 = local read "Maker"() -> (w509:string)
        n134 = Format Into String(format string="WHERE PART_NAME='%s' AND PRODUCT='%s' " ("condition"), w507, w508) -> (resulting string=w527:string)  [unwired: 2 in, 1 out]
        n135 = Format Into String(format string="WHERE MAKER='%s' AND PRODUCT='%s' AND PART_NAME='%s'" ("condition"), w509, w508, w507) -> (resulting string=w520:string)  [unwired: 2 in, 1 out]
        n136 = call <vilib>:"DB Tools Select Data.vi"("condition"=w527, "columns"=string[] ["DISTINCT MAKER"], "table"=w510, "connection reference"=w525) -> ("data"=w529:variant[][], "connection reference out"=w511:T1)  [unwired: 2 in, 1 out]
        n137 = call <vilib>:"DB Tools Select Data.vi"("condition"=w520, "columns"=string[] ["`LENGTH-OFFSET`"], "table"=w510, "connection reference"=w511) -> ("data"=w523:variant[][])  [unwired: 2 in, 2 out]
        n138 = xnode "Database Variant To Data"("database variant"=w529, "type"=string[][] []) -> ("data"=w532:string[][])  [unwired: 1 in, 1 out]
        n139 = xnode "Database Variant To Data"("database variant"=w523, "type"=string[][] []) -> ("data"=w518:string[][])  [unwired: 1 in, 1 out]
        n140 = Index Array(array=w532, index (col)=0 ("index (row)")) -> (element=w524:string[])  [unwired: 1 in]
        n141 = for {
          tunnel: w518 -> [w536] mode=indexing
          tunnel: [w534] -> w517
          stop <- w533 continue-if-true
          n142 = Index Array(array=w536, index=0 ("index (row)")) -> (element=w534:string)
          n143 = Empty String/Path?(string/path=w534) -> (empty?=w533:bool)
        }
        n144 = property on="Maker" class="CmbBox"("Strings[]"=w524) -> ()  [unwired: 2 in, 2 out]
        n145 = Match Pattern(string=w517, regular expression="-") -> (before substring=w515:string, after substring=w514:string)  [unwired: 1 in, 2 out]
        n146 = Decimal String To Number(string=w515) -> (number=w512:i32)  [unwired: 2 in, 1 out]
        n147 = Decimal String To Number(string=w514) -> (number=w513:i32)  [unwired: 2 in, 1 out]
        n148 = local write "Length"(w512) -> ()
        n149 = local write "Offset"(w513) -> ()
      }
      event "Maker": Value Change {
        n150 = event-data() -> ()  [unwired: 1 in, 6 out]
        n151 = local write "Lot Maker"("" ("Lot Maker")) -> ()
        n152 = local read "Part Name"() -> (w635:string)
        n153 = local read "Product"() -> (w636:string)
        n154 = local read "Maker"() -> (w637:string)
        n155 = Format Into String(format string="WHERE MAKER='%s' AND PRODUCT='%s' AND PART_NAME='%s'" ("condition"), w637, w636, w635) -> (resulting string=w634:string)  [unwired: 2 in, 1 out]
        n156 = Format Into String(format string="WHERE MAKER='%s' AND PRODUCT='%s' " ("condition"), w637, w636) -> (resulting string=w646:string)  [unwired: 2 in, 1 out]
        n157 = call <vilib>:"DB Tools Select Data.vi"("condition"=w646, "columns"=string[] ["DISTINCT PART_NAME"], "table"=w640, "connection reference"=w644) -> ("data"=w648:variant[][], "connection reference out"=w641:T1)  [unwired: 2 in, 1 out]
        n158 = call <vilib>:"DB Tools Select Data.vi"("condition"=w634, "columns"=string[] ["`LENGTH-OFFSET`"], "table"=w640, "connection reference"=w641) -> ("data"=w642:variant[][])  [unwired: 2 in, 2 out]
        n159 = xnode "Database Variant To Data"("database variant"=w648, "type"=string[][] []) -> ("data"=w651:string[][])  [unwired: 1 in, 1 out]
        n160 = Index Array(array=w651, index (col)=0 ("index (row)")) -> (element=w643:string[])  [unwired: 1 in]
        n161 = xnode "Database Variant To Data"("database variant"=w642, "type"=string[][] []) -> ("data"=w632:string[][])  [unwired: 1 in, 1 out]
        n162 = for {
          tunnel: w632 -> [w655] mode=indexing
          tunnel: [w653] -> w631
          stop <- w652 continue-if-true
          n163 = Index Array(array=w655, index=0 ("index (row)")) -> (element=w653:string)
          n164 = Empty String/Path?(string/path=w653) -> (empty?=w652:bool)
        }
        n165 = property on="Part Name" class="CmbBox"("Strings[]"=w643) -> ()  [unwired: 2 in, 2 out]
        n166 = Match Pattern(string=w631, regular expression="-") -> (before substring=w629:string, after substring=w628:string)  [unwired: 1 in, 2 out]
        n167 = Decimal String To Number(string=w629) -> (number=w626:i32)  [unwired: 2 in, 1 out]
        n168 = Decimal String To Number(string=w628) -> (number=w627:i32)  [unwired: 2 in, 1 out]
        n169 = local write "Length"(w626) -> ()
        n170 = local write "Offset"(w627) -> ()
      }
      event "Barcode (F1)", "Part No (F2)": Value Change {
        n171 = event-data() -> ("NewVal"=w755:string)  [unwired: 1 in, 5 out]
        n172 = local read "Barcode (F1)"() -> (w763:string)
        n173 = Empty String/Path?(string/path=w763) -> (empty?=w744:bool)
        n174 = local read "Offset"() -> (w753:dbl)
        n175 = local read "Length"() -> (w754:dbl)
        n176 = Less Or Equal To 0?(x=w754) -> (x <= 0?=w757:bool)
        n177 = String Length(string=w755) -> (length=w756:i32)
        n178 = Select(t=w756, s=w757, f=w754) -> (s? t:f=w745:dbl)
        n179 = String Subset(string=w755, offset (0)=w753, length (rest)=w745) -> (substring=w752:string)
        n180 = case shown="True" w744 {
          tunnel: [w805 w813] -> w776
          tunnel: w752 -> [_ w809]
          frame True {
            n181 = local read "Part No (F2)"() -> (w802:string)
            n182 = local read "Part Name"() -> (w806:string)
            n183 = local read "Product"() -> (w803:string)
            n184 = local read "Maker"() -> (w804:string)
            n185 = Format Into String(format string="WHERE MAKER='%s' AND PRODUCT='%s' AND PART_NAME='%s' AND PART_NO='%s'" ("condition"), w804, w803, w806, w802) -> (resulting string=w805:string)  [unwired: 2 in, 1 out]
          }
          frame False {
            w810 = "%"
            n186 = Concatenate Strings(w810, w809, w810) -> (w808:string)
            n187 = local read "Part Name"() -> (w814:string)
            n188 = local read "Product"() -> (w811:string)
            n189 = local read "Maker"() -> (w812:string)
            n190 = Format Into String(format string="WHERE MAKER='%s' AND PRODUCT='%s' AND PART_NAME='%s' AND BARCODE LIKE '%s'" ("condition"), w812, w811, w814, w808) -> (resulting string=w813:string)  [unwired: 2 in, 1 out]
          }
        }
        n191 = call <vilib>:"DB Tools Select Data.vi"("condition"=w776, "table"=w774, "connection reference"=w775) -> ("data"=w777:variant[][])  [unwired: 3 in, 2 out]
        n192 = xnode "Database Variant To Data"("database variant"=w777, "type"=T6[] []) -> ("data"=w772:T6[])  [unwired: 1 in, 1 out]
        n193 = local read "Offset"() -> (w749:dbl)
        n194 = local read "Table"() -> (w762:string[][])
        n195 = Index Array(array=w772, index=0) -> (element=w770:T6)
        n196 = Unbundle By Name(w770) -> ("BARCODE"=w748:string, "PART_NO"=w769:string, "LOT_SIZE"=w767:dbl, "UNIT"=w766:string, "LENGTH-OFFSET"=w768:string, "ITEM_CODE"=w758:string, "PART_NO"=w765:string, "INVENTORY_LOCAL"=w764:string)
        n197 = local read "Barcode (F1)"() -> (w747:string)
        n198 = Index Array(array=w762, index (col)=1 ("disabled index (col)")) -> (element=w760:string[])  [unwired: 1 in]
        n199 = String Subset(string=w747, offset (0)=w749, length (rest)=w745) -> (substring=w750:string)
        n200 = String Subset(string=w748, offset (0)=w749, length (rest)=w745) -> (substring=w751:string)
        n201 = Equal?(x=w750, y=w751) -> (x = y?=w746:bool)
        n202 = Search 1D Array(1D array=w760, element=w758) -> (index of element=w759:i32)  [unwired: 1 in]
        n203 = local write "Item Code (F3)"(w758) -> ()
        n204 = case shown="-1" w759 {
          tunnel: w769 -> [w787 _]
          tunnel: w768 -> [w786 _]
          tunnel: w767 -> [w785 _]
          tunnel: w766 -> [w784 _]
          tunnel: w765 -> [w783 _]
          tunnel: w764 -> [w782 _]
          tunnel: w748 -> [w781 _]
          tunnel: w758 -> [_ w798]
          tunnel: w746 -> [w779 _]
          tunnel: w744 -> [w778 _]
          frame 0, Default {
            n205 = Or(x=w779, y=w778) -> (x .or. y?=w780:bool)
            n206 = case shown="False" w780 {
              tunnel: w787 -> [w792 _]
              tunnel: w786 -> [_ _]
              tunnel: w785 -> [w791 _]
              tunnel: w784 -> [w790 _]
              tunnel: w783 -> [w789 _]
              tunnel: w782 -> [w788 _]
              tunnel: w781 -> [_ _]
              frame True {
                n207 = local write "Unit 2"(w790) -> ()
                n208 = local write "Unit"(w790) -> ()
                n209 = local write "Quantity"(w791) -> ()
                n210 = local write "Part No (F2)"(w792) -> ()
                n211 = local write "Lot Size"(w791) -> ()
                n212 = local write "Maker Code"(w789) -> ()
                n213 = local write "Location"(w788) -> ()
              }
              frame False {
                w793 = 0
                w794 = ""
                n214 = local write "Unit 2"(w794) -> ()
                n215 = local write "Unit"(w794) -> ()
                n216 = local write "Quantity"(w793) -> ()
                n217 = local write "Part No (F2)"(w794) -> ()
                n218 = local write "Lot Size"(w793) -> ()
                n219 = local write "Maker Code"(w794) -> ()
                n220 = local write "Location"(w794) -> ()
              }
            }
          }
          frame -1 {
            n221 = local write "Item Code (F3)"("" ("Item Code")) -> ()
            n222 = Concatenate Strings(w798, "  doesn't exist in INVOICE.\nPlease check again!" ("message")) -> (w797:string)
            n223 = One Button Dialog(message=w797) -> (true=w796:bool)  [unwired: 1 in]
            n224 = flat-sequence {
              tunnel: [w801] -> w795
              tunnel: w796 -> [w801]
              frame #0 {
              }
            }
            n225 = property on="Barcode (F1)" class="Str"("Key Focus"=w795) -> ()  [unwired: 2 in, 2 out]
          }
        }
      }
      event "Barcode (F1)", "Part No (F2)": Mouse Down? {
        w1229 = 0
        w1230 = ""
        n226 = event-data() -> ()  [unwired: 1 in, 8 out]
        n227 = local write "Quantity"(w1229) -> ()
        n228 = local write "Amount (F4)"(w1229) -> ()
        n229 = local write "Lot Size"(w1229) -> ()
        n230 = local write "Unit"(w1230) -> ()
        n231 = local write "Unit 2"(w1230) -> ()
        n232 = local write "Part No (F2)"(w1230) -> ()
        n233 = local write "Item Code (F3)"(w1230) -> ()
        n234 = local write "Maker Code"(w1230) -> ()
        n235 = local write "Location"(w1230) -> ()
        n236 = local write "Barcode (F1)"(w1230) -> ()
        n237 = event-data() -> ()  [unwired: 2 in, 1 out]
      }
      event "BUTTON_INPUT": Value Change {
        n238 = event-data() -> ("OldVal"=w1231:bool)  [unwired: 1 in, 5 out]
        n239 = flat-sequence {
          tunnel: [w1267] -> w1232
          tunnel: w1231 -> [w1267]
          frame #0 {
            n240 = Wait (ms)(milliseconds to wait=u32 500) -> ()  [unwired: 1 out]
          }
        }
        n241 = local write "BUTTON_INPUT"(w1232) -> ()
        n242 = local read "Item Code (F3)"() -> (w1260:string)
        n243 = local read "Amount (F4)"() -> (w1254:dbl)
        n244 = local read "Maker Code"() -> (w1259:string)
        n245 = local read "Part No (F2)"() -> (w1261:string)
        n246 = local read "Part Name"() -> (w1263:string)
        n247 = local read "Input Date"() -> (w1266:timestamp)
        n248 = local read "Input No."() -> (w1237:string)
        n249 = local read "Quantity"() -> (w1255:dbl)
        n250 = local read "Product"() -> (w1264:string)
        n251 = local read "Lot Size"() -> (w1258:dbl)
        n252 = local read "ECODE"() -> (w1236:string)
        n253 = local read "Maker"() -> (w1262:string)
        n254 = local read "Unit 2"() -> (w1256:string)
        n255 = local read "Unit"() -> (w1257:string)
        n256 = Less?(x=w1266, y=timestamp(3345127200 s since 1904-01-01)) -> (x < y?=w1252:bool)
        n257 = Empty String/Path?(string/path=w1264) -> (empty?=w1251:bool)
        n258 = Empty String/Path?(string/path=w1263) -> (empty?=w1250:bool)
        n259 = Empty String/Path?(string/path=w1262) -> (empty?=w1249:bool)
        n260 = Empty String/Path?(string/path=w1261) -> (empty?=w1248:bool)
        n261 = Empty String/Path?(string/path=w1260) -> (empty?=w1247:bool)
        n262 = Empty String/Path?(string/path=w1259) -> (empty?=w1246:bool)
        n263 = Empty String/Path?(string/path=w1237) -> (empty?=w1253:bool)
        n264 = Empty String/Path?(string/path=w1257) -> (empty?=w1244:bool)
        n265 = Empty String/Path?(string/path=w1256) -> (empty?=w1243:bool)
        n266 = Empty String/Path?(string/path=w1236) -> (empty?=w1235:bool)
        n267 = Less Or Equal To 0?(x=w1258) -> (x <= 0?=w1245:bool)
        n268 = Less Or Equal To 0?(x=w1255) -> (x <= 0?=w1242:bool)
        n269 = Less Or Equal To 0?(x=w1254) -> (x <= 0?=w1241:bool)
        n270 = Compound Arithmetic op=OR(w1253, w1252, w1251, w1250, w1249, w1248, w1247, w1246, w1245, w1244, w1243, w1242, w1241, w1235) -> (w1240:bool)
        n271 = case shown="True" w1240 {
          tunnel: w1239 -> [w1291 _]
          tunnel: w1238 -> [w1278 _]
          tunnel: w1237 -> [w1290 _]
          tunnel: [TRUE FALSE ("Key Focus")] -> w1234
          frame False {
            n272 = Format Into String(format string="`%s`.`STORE_INPUT_%s`", w1278, w1290) -> (resulting string=w1279:string)  [unwired: 2 in, 1 out]
            n273 = call <vilib>:"DB Tools Select Data.vi"("table"=w1279, "connection reference"=w1291) -> ("error out"=w1289:errorcluster, "data"=w1287:variant[][], "connection reference out"=w1281:T1)  [unwired: 4 in]
            n274 = xnode "Database Variant To Data"("database variant"=w1287, "error in (no error)"=w1289, "type"=T3[] []) -> ("data"=w1282:T3[])  [unwired: 1 out]
            n275 = xnode "Database Variant To Data"("database variant"=w1287, "type"=string[][] []) -> ("data"=w1276:string[][])  [unwired: 1 in, 1 out]
            n276 = local write "Table"(w1276) -> ()
            n277 = local read "Item Code (F3)"() -> (w1277:string)
            n278 = Index Array(array=w1276, index (col)=1 ("disabled index (col)")) -> (element=w1284:string[])  [unwired: 1 in]
            n279 = Search 1D Array(1D array=w1284, element=w1277) -> (index of element=w1283:i32)  [unwired: 1 in]
            n280 = case shown="0, Default" w1283 {
              selector: w1283 -> [w1299 _]
              tunnel: w1282 -> [w1304 _]
              tunnel: w1281 -> [w1301 _]
              tunnel: w1279 -> [w1300 _]
              tunnel: w1278 -> [w1303 _]
              tunnel: w1277 -> [w1302 _]
              frame 0, Default {
                w1293 = 0  # number copy to print
                n281 = local read "Amount (F4)"() -> (w1298:dbl)
                n282 = for {
                  N: w1298 -> [_]
                  tunnel: w1303 -> [w1349]
                  tunnel: w1302 -> [w1348]
                  tunnel: w1301 -> [w1345]
                  tunnel: w1300 -> [w1344]
                  tunnel: w1299 -> [w1341]
                  shift-right: [w1335] -> _
                  shift-left: w1304 -> [w1334]
                  tunnel: [w1333] -> w1295 mode=indexing
                  shift-right: [w1331] -> w1292
                  shift-left: w1293 -> [w1332]
                  stop <- w1336 stop-if-true
                  n283 = Index Array(array=w1334, index=w1341) -> (element=w1347:T3)
                  n284 = Unbundle By Name(w1347) -> ("ITEM_CODE"=w1343:string, "QUANTITY"=w1339:dbl, "BALANCE"=w1338:dbl, "INVOICE_NO"=w1346:string)  [unwired: 6 out]
                  n285 = Bundle By Name(cluster=T2 {"Row"=0, "Column"=0} ("Index Values"), "Row"=w1341) -> (w1342:T2)
                  n286 = property on="Table" class="Tbl (strict)"("Index Values"=w1342) -> ()  [unwired: 2 in, 2 out]
                  n287 = Less Than 0?(x=w1338) -> (x < 0?=w1337:bool)
                  n288 = case shown="True" w1337 {
                    tunnel: w1349 -> [_ w1396]
                    tunnel: w1348 -> [_ w1395]
                    tunnel: w1346 -> [_ w1384]
                    tunnel: w1345 -> [_ w1379]
                    tunnel: w1344 -> [_ w1374]
                    tunnel: w1343 -> [_ w1367]
                    tunnel: w1339 -> [_ w1364]
                    tunnel: [w1352 _] -> w1336
                    tunnel: [w1351 w1360] -> w1335
                    tunnel: w1334 -> [w1351 _]
                    tunnel: [_ w1356] -> w1333
                    tunnel: w1332 -> [w1350 w1355]
                    tunnel: [w1350 w1354] -> w1331
                    frame False {
                      n289 = One Button Dialog(message="Quantity is Enough!") -> (true=w1352:bool)  [unwired: 1 in]
                    }
                    frame True {
                      w1357 = "" ("OUTPUT_NO")
                      w1358 = timestamp(0 s since 1904-01-01) ("OUTPUT_DATE")
                      n290 = Format Into String(format string="`%s`.`%s`", w1396, w1395) -> (resulting string=w1393:string)  [unwired: 2 in, 1 out]
                      n291 = Increment(x=w1355) -> (x+1=w1354:i32)
                      n292 = local read "Input Date"() -> (w1390:timestamp)
                      n293 = local read "Lot Maker"() -> (w1391:string)
                      n294 = local read "Quantity"() -> (w1378:dbl)
                      n295 = call <vilib>:"DB Tools List Columns.vi"("table"=w1393, "connection reference"=w1379) -> ("columns"=w1394:string[])  [unwired: 2 in, 3 out]
                      n296 = local read "ECODE"() -> (w1359:string)
                      n297 = Empty Array?(array=w1394) -> (empty?=w1380:bool)
                      n298 = case shown="True" w1380 {
                        tunnel: w1379 -> [w1869 w1871]
                        tunnel: w1393 -> [w1868 w1870]
                        tunnel: [w1868 w1870] -> w1386
                        tunnel: [w1869 w1872] -> w1389
                        frame False {
                        }
                        frame True {
                          n299 = Format Into String(format string="CREATE TABLE %s (\n  `ITEM_CODE` VARCHAR(50) NOT NULL COMMENT '',\n  `INVOICE_NO` VARCHAR(1000) NULL COMMENT '',\n  `INVOICE_DATE` DATETIME NULL COMMENT '',\n  `LOT_MAKER` VARCHAR(100) NULL COMMENT '',\n  `QUANTITY` DOUBLE NULL COMMENT '',\n  `INVOICE_ECODE` VARCHAR(20) NULL COMMENT '',\n  `INPUT_NO` VARCHAR(1000) NULL COMMENT '',\n  `INPUT_DATE` DATETIME NULL COMMENT '',\n  `INPUT_ECODE` VARCHAR(20) NULL COMMENT '',\n  `LINEBACK_NO` VARCHAR(1000) NULL COMMENT '',\n  `LINEBACK_DATE` DATETIME NULL COMMENT '',\n  `LINEBACK_ECODE` VARCHAR(20) NULL COMMENT '',\n  `OUTPUT_NO` VARCHAR(1000) NULL COMMENT '',\n  `OUTPUT_DATE` DATETIME NULL COMMENT '',\n  `OUTPUT_ECODE` VARCHAR(20) NULL COMMENT '',\n  `DESTINATION` VARCHAR(1000) NULL COMMENT '');\n", w1870) -> (resulting string=w1873:string)  [unwired: 2 in, 1 out]
                          n300 = call-poly <vilib>:"DB Tools Execute Query.vi"("SQL query"=w1873, "connection reference"=w1871) -> ("error out"=w1876:errorcluster, "recordset reference"=w1875:T10)  [unwired: 6 in]
                          n301 = call-poly <vilib>:"DB Tools Free Object.vi"("error in (no error)"=w1876, "recordset reference"=w1875) -> ("connection reference"=w1872:T1)  [unwired: 8 in, 1 out]
                        }
                      }
                      n302 = Format Into String(format string="WHERE ITEM_CODE='%s'" ("condition"), w1367) -> (resulting string=w1369:string)  [unwired: 2 in, 1 out]
                      n303 = Format Into String(format string="WHERE INPUT_NO='%s'" ("condition"), w1384) -> (resulting string=w1383:string)  [unwired: 2 in, 1 out]
                      n304 = Bundle By Name(cluster=T8 {"ITEM_CODE"="", "INVOICE_NO"="", "INVOICE_DATE"=timestamp(0 s since 1904-01-01), "LOT_MAKER"="", "QUANTITY"=0.0, "INVOICE_ECODE"="", "INPUT_NO"="", "INPUT_DATE"=timestamp(0 s since 1904-01-01), "INPUT_ECODE"="", "LINEBACK_NO"="", "LINEBACK_DATE"=timestamp(0 s since 1904-01-01), "LINEBACK_ECODE"="", "OUTPUT_NO"="", "OUTPUT_DATE"=timestamp(0 s since 1904-01-01), "OUTPUT_ECODE"="", "DESTINATION"=""}, "ITEM_CODE"=w1367, "INVOICE_NO"=w1384, "INVOICE_DATE"=w1390, "LOT_MAKER"=w1391, "QUANTITY"=w1378, "INPUT_NO"=w1384, "INPUT_DATE"=w1390, "INPUT_ECODE"=w1359, "INVOICE_ECODE"=w1359, "LINEBACK_NO"=w1357, "LINEBACK_DATE"=w1358, "LINEBACK_ECODE"=w1357, "OUTPUT_NO"=w1357, "OUTPUT_DATE"=w1358, "OUTPUT_ECODE"=w1357, "DESTINATION"=w1357) -> (w1388:T8)
                      n305 = call <vilib>:"DB Tools Insert Data.vi"("data"=w1388, "table"=w1386, "connection reference"=w1389) -> ("error out"=w1356:errorcluster, "connection reference out"=w1387:T1)  [unwired: 7 in]
                      n306 = call <vilib>:"DB Tools Select Data.vi"("condition"=w1383, "columns"=string[] ["QUANTITY"], "table"=w1386, "connection reference"=w1387) -> ("data"=w1381:variant[][], "connection reference out"=w1375:T1)  [unwired: 2 in, 1 out]
                      n307 = xnode "Database Variant To Data"("database variant"=w1381, "type"=dbl[][] []) -> ("data"=w1371:dbl[][])  [unwired: 1 in, 1 out]
                      n308 = Add Array Elements(numeric array=w1371) -> (sum=w1363:dbl)
                      n309 = Subtract(x=w1363, y=w1364) -> (x-y=w1366:dbl)
                      n310 = Bundle(w1363, w1366) -> (w1365:cluster{dbl, dbl})  [unwired: 1 in]
                      n311 = call <vilib>:"DB Tools Update Data.vi"("condition"=w1369, "data"=w1365, "columns"=string[] ["INPUT", "BALANCE"], "table"=w1374, "connection reference"=w1375) -> ("connection reference out"=w1368:T1)  [unwired: 5 in, 1 out]
                      n312 = call <vilib>:"DB Tools Select Data.vi"("table"=w1374, "connection reference"=w1368) -> ("data"=w1362:variant[][])  [unwired: 4 in, 2 out]
                      n313 = xnode "Database Variant To Data"("database variant"=w1362, "type"=T3[] []) -> ("data"=w1360:T3[])  [unwired: 1 in, 1 out]
                      n314 = xnode "Database Variant To Data"("database variant"=w1362, "type"=string[][] []) -> ("data"=w1376:string[][])  [unwired: 1 in, 1 out]
                      n315 = local write "Table"(w1376) -> ()
                    }
                  }
                }
                n316 = local read "AUTO_PRINT"() -> (w1294:bool)
                n317 = Or Array Elements(Boolean array=w1295) -> (logical OR=w1297:bool)
                n318 = case shown="False" w1297 {
                  tunnel: ["SUCCESSFUL!!" "ERROR when input"] -> w1296
                  frame False {
                  }
                  frame True {
                  }
                }
                n319 = case shown="True" w1294 {
                  tunnel: w1292 -> [_ w1319]
                  frame False {
                  }
                  frame True {
                    w1323 = "\\" ("string")
                    n320 = local read "Maker Code"() -> (w1311:string)
                    n321 = call <vilib>:"Space Constant.vi"() -> ("String"=w1322:string)
                    n322 = local read "Input Date"() -> (w1326:timestamp)
                    n323 = local read "Unit 2"() -> (w1321:string)
                    n324 = local read "Lot Maker"() -> (w1316:string)
                    n325 = local read "Maker"() -> (w1312:string)
                    n326 = local read "Location"() -> (w1310:string)
                    n327 = Format Date/Time String(time format string (%c)="%d/%m/%Y", seconds (now)=w1326) -> (date/time string=w1314:string)  [unwired: 1 in]
                    n328 = local read "Input No."() -> (w1313:string)
                    n329 = local read "Quantity"() -> (w1324:dbl)
                    n330 = Number To Decimal String(number=w1324) -> (decimal integer string=w1308:string)  [unwired: 1 in]
                    n331 = Concatenate Strings(w1308, w1322, w1321) -> (w1307:string)
                    n332 = local read "Item Code (F3)"() -> (w1315:string)
                    n333 = local read "Product"() -> (w1309:string)
                    n334 = local read "ECODE"() -> (w1306:string)
                    n335 = Concatenate Strings(w1315, w1323, w1314, w1323, w1313, w1323, w1308, w1323, w1316) -> (w1317:string)
                    n336 = Bundle By Name(cluster=T7 {"QR_code Text"="", "Lot Maker"="", "Item Code (F3)"="", "date/time string"="", "Invoice No."="", "Maker"="", "Part No.(F2) "="", "Location"="", "Product"="", "Qty"="", "ECODE"=""} ("output cluster"), "QR_code Text"=w1317, "Lot Maker"=w1316, "Item Code (F3)"=w1315, "date/time string"=w1314, "Invoice No."=w1313, "Maker"=w1312, "Part No.(F2)"=w1311, "Location"=w1310, "Product"=w1309, "Qty"=w1307, "ECODE"=w1306) -> (w1305:T7)
                    n337 = call "QR Code Generator Main.vi"("number of copies (1)"=w1319, "Print Button"=TRUE, "output cluster"=w1305) -> ()  [unwired: 9 in]
                  }
                }
                n338 = flat-sequence {
                  tunnel: w1296 -> [w1327]
                  frame #0 {
                    n339 = One Button Dialog(message=w1327) -> ()  [unwired: 1 in, 1 out]
                  }
                  frame #1 {
                    n340 = Wait (ms)(milliseconds to wait=u32 10) -> ()  [unwired: 1 out]
                  }
                }
              }
              frame -1 {
                n341 = One Button Dialog(message="Item code is wrong!\nPlease Check again") -> ()  [unwired: 1 in, 1 out]
              }
            }
          }
          frame True {
            n342 = flat-sequence {
              tunnel: "Fill all data, Please! \nQuantity >0" ("message") -> [w2309]
              tunnel: [TRUE ("Key Focus")] -> w2305
              tunnel: w2305 -> [w2311]
              tunnel: [w2311] -> w2304
              tunnel: w2304 -> [w2312]
              frame #0 {
                n343 = One Button Dialog(message=w2309) -> ()  [unwired: 1 in, 1 out]
              }
              frame #1 {
                n344 = Wait (ms)(milliseconds to wait=u32 10) -> ()  [unwired: 1 out]
              }
              frame #2 {
                n345 = property on="Barcode (F1)" class="Str"("Key Focus"=w2312) -> ()  [unwired: 2 in, 2 out]
              }
            }
          }
        }
        n346 = flat-sequence {
          tunnel: [w1270] -> w1233
          tunnel: w1234 -> [w1270]
          frame #0 {
            n347 = Wait (ms)(milliseconds to wait=u32 10) -> ()  [unwired: 1 out]
          }
        }
        n348 = case shown="False" w1233 {
          frame False {
          }
          frame True {
            w1273 = ""
            w1274 = 0.0
            n349 = local write "Lot Size"(w1274) -> ()
            n350 = local write "Amount (F4)"(w1274) -> ()
            n351 = local write "Quantity"(w1274) -> ()
            n352 = local write "Unit"(w1273) -> ()
            n353 = local write "Unit 2"(w1273) -> ()
            n354 = property on="Barcode (F1)" class="Str"("Key Focus"=TRUE) -> ()  [unwired: 2 in, 2 out]
            n355 = property on="Excle Path (F1)" class="Path"("Visible"=FALSE) -> ()  [unwired: 2 in, 2 out]
            n356 = local write "Part No (F2)"(w1273) -> ()
            n357 = local write "Item Code (F3)"(w1273) -> ()
            n358 = local write "Maker Code"(w1273) -> ()
            n359 = local write "Barcode (F1)"(w1273) -> ()
            n360 = local write "Location"(w1273) -> ()
          }
        }
      }
      event "PRINT button": Value Change {
        n361 = event-data() -> ("OldVal"=w2314:bool)  [unwired: 1 in, 5 out]
        n362 = local read "Input Date"() -> (w2331:timestamp)
        n363 = local read "Item Code (F3)"() -> (w2335:string)
        n364 = local read "Amount (F4)"() -> (w2336:dbl)
        n365 = local read "ECODE"() -> (w2334:string)
        n366 = local read "Maker Code"() -> (w2326:string)
        n367 = local read "Maker"() -> (w2327:string)
        n368 = local read "Quantity"() -> (w2325:dbl)
        n369 = local read "Unit 2"() -> (w2328:string)
        n370 = flat-sequence {
          tunnel: [w2339] -> w2313
          tunnel: w2314 -> [w2339]
          frame #0 {
            n371 = Wait (ms)(milliseconds to wait=u32 500) -> ()  [unwired: 1 out]
          }
        }
        n372 = Format Date/Time String(time format string (%c)="%d/%m/%Y", seconds (now)=w2331) -> (date/time string=w2333:string)  [unwired: 1 in]
        n373 = Less?(x=w2331, y=timestamp(3345170400 s since 1904-01-01)) -> (x < y?=w2320:bool)
        n374 = local read "Product"() -> (w2329:string)
        n375 = local read "Input No."() -> (w2332:string)
        n376 = Empty String/Path?(string/path=w2334) -> (empty?=w2323:bool)
        n377 = Empty String/Path?(string/path=w2335) -> (empty?=w2324:bool)
        n378 = Empty String/Path?(string/path=w2326) -> (empty?=w2316:bool)
        n379 = Empty String/Path?(string/path=w2328) -> (empty?=w2319:bool)
        n380 = Empty String/Path?(string/path=w2327) -> (empty?=w2318:bool)
        n381 = Empty String/Path?(string/path=w2329) -> (empty?=w2321:bool)
        n382 = local write "PRINT button"(w2313) -> ()
        n383 = Empty String/Path?(string/path=w2332) -> (empty?=w2322:bool)
        n384 = Less Or Equal To 0?(x=w2325) -> (x <= 0?=w2317:bool)
        n385 = Compound Arithmetic op=OR(w2324, w2323, w2322, w2321, w2320, w2319, w2318, w2317, w2316) -> (w2315:bool)
        n386 = case shown="False" w2315 {
          tunnel: w2326 -> [w2344 _]
          tunnel: w2327 -> [w2345 _]
          tunnel: w2328 -> [w2355 _]
          tunnel: w2335 -> [w2348 _]
          tunnel: w2334 -> [w2341 _]
          tunnel: w2333 -> [w2347 _]
          tunnel: w2332 -> [w2346 _]
          tunnel: w2329 -> [w2343 _]
          tunnel: w2325 -> [w2354 _]
          tunnel: w2336 -> [w2353 _]
          frame False {
            w2359 = "\\" ("string")
            n387 = call <vilib>:"Space Constant.vi"() -> ("String"=w2358:string)
            n388 = local read "Lot Maker"() -> (w2349:string)
            n389 = Number To Decimal String(number=w2354) -> (decimal integer string=w2357:string)  [unwired: 1 in]
            n390 = Concatenate Strings(w2357, w2358, w2355) -> (w2342:string)
            n391 = local read "Location"() -> (w2350:string)
            n392 = Concatenate Strings(w2348, w2359, w2347, w2359, w2346, w2359, w2357, w2359, w2349) -> (w2351:string)
            n393 = Bundle By Name(cluster=T7 {"QR_code Text"="", "Lot Maker"="", "Item Code (F3)"="", "date/time string"="", "Invoice No."="", "Maker"="", "Part No.(F2) "="", "Location"="", "Product"="", "Qty"="", "ECODE"=""} ("output cluster"), "QR_code Text"=w2351, "Lot Maker"=w2349, "Item Code (F3)"=w2348, "date/time string"=w2347, "Invoice No."=w2346, "Maker"=w2345, "Part No.(F2)"=w2344, "Location"=w2350, "Product"=w2343, "Qty"=w2342, "ECODE"=w2341) -> (w2340:T7)
            n394 = call "QR Code Generator Main.vi"("number of copies (1)"=w2353, "Print Button"=TRUE, "output cluster"=w2340) -> ()  [unwired: 9 in]
          }
          frame True {
            n395 = One Button Dialog(message="Full fill Data, Please") -> ()  [unwired: 1 in, 1 out]
          }
        }
      }
      event "BUTTON_ADD": Value Change {
        n396 = event-data() -> ("OldVal"=w2365:bool)  [unwired: 1 in, 5 out]
        n397 = local write "BUTTON_ADD"(w2365) -> ()
        n398 = local read "ECODE"() -> (w2361:string)
        n399 = call "Login.vi"("connection reference"=w2362, "ACCOUNT:"=w2361, "Permission"=string[] ["Manager", "Leader"]) -> ("OK"=w2363:bool)  [unwired: 7 in, 1 out]
        n400 = case shown="True" w2363 {
          tunnel: w2362 -> [_ w2387]
          frame False {
          }
          frame True {
            w2369 = 0.0 ("TARE")
            n401 = local read "Barcode (F1)"() -> (w2372:string)
            n402 = local read "Item Code (F3)"() -> (w2384:string)
            n403 = local read "Part No (F2)"() -> (w2381:string)
            n404 = local read "Location"() -> (w2371:string)
            n405 = local read "Part Name"() -> (w2383:string)
            n406 = local read "Length"() -> (w2377:dbl)
            n407 = local read "Offset"() -> (w2378:dbl)
            n408 = local read "Lot Size"() -> (w2380:dbl)
            n409 = local read "Unit"() -> (w2379:string)
            n410 = local read "Maker"() -> (w2382:string)
            n411 = local read "Product"() -> (w2385:string)
            n412 = Number To Decimal String(number=w2378) -> (decimal integer string=w2374:string)  [unwired: 1 in]
            n413 = Number To Decimal String(number=w2377) -> (decimal integer string=w2375:string)  [unwired: 1 in]
            n414 = Concatenate Strings(w2375, "-" ("string"), w2374) -> (w2373:string)
            n415 = Bundle By Name(cluster=T9 {"PRODUCT"="", "ITEM CODE"="", "PART NAME"="", "MAKER"="", "PART NO"="", "LOT SIZE"=0.0, "UNIT"="", "LENGTH-OFFSET"="", "BARCODE"="", "PROCESS"="", "INVENTORY LOCAL"="", "TARE"=0.0, "SAMPLE"=0.0} ("ITEM_DATA"), "PRODUCT"=w2385, "ITEM CODE"=w2384, "PART NAME"=w2383, "MAKER"=w2382, "PART NO"=w2381, "LOT SIZE"=w2380, "UNIT"=w2379, "LENGTH-OFFSET"=w2373, "BARCODE"=w2372, "PROCESS"="", "INVENTORY LOCAL"=w2371, "TARE"=w2369, "SAMPLE"=w2369) -> (w2366:T9)
            n416 = call "Import_Source_Item_Code.vi"("CONTROL Control"=enum32{"IMPRORT", "ADD"}."ADD", "UPDATE ONLY"=FALSE, "ITEM_DATA"=w2366, "connection reference"=w2387) -> ()  [unwired: 8 in]
          }
        }
      }
      event Timeout {
        (unwired) 1 ("disabled index (col)")
        n417 = event-data() -> ()  [unwired: 1 in, 3 out]
        n418 = local read "Input No."() -> (w2393:string)
        n419 = Format Into String(format string="`%s`.`STORE_INPUT_%s`", w2394, w2393) -> (resulting string=w2389:string)  [unwired: 2 in, 1 out]
        n420 = call <vilib>:"DB Tools Select Data.vi"("table"=w2389, "connection reference"=w2395) -> ("data"=w2392:variant[][])  [unwired: 4 in, 2 out]
        n421 = xnode "Database Variant To Data"("database variant"=w2392, "type"=string[][] []) -> ("data"=w2388:string[][])  [unwired: 1 in, 1 out]
        n422 = local write "Table"(w2388) -> ()
      }
      event "Search": Value Change {
        n423 = event-data() -> ("NewVal"=w2440:string)  [unwired: 1 in, 5 out]
        n424 = local read "Table"() -> (w2447:string[][])
        n425 = Index Array(array=w2447, index (col)=1 ("disabled index (col)")) -> (element=w2445:string[])  [unwired: 1 in]
        n426 = for {
          tunnel: w2445 -> [w2455] mode=indexing
          tunnel: w2440 -> [w2454]
          shift-right: [w2452] -> w2442
          shift-left: i32[] [] ("Find Array") -> [w2451]
          shift-right: [w2448] -> _
          shift-left: 0 -> [w2449]
          i -> [w2450]
          n427 = Search and Replace String(input string=w2455, search string=w2454, replace string=w2454) -> (number of replacements=w2453:i32)  [unwired: 5 in, 3 out]
          n428 = case shown="0" w2453 {
            tunnel: [w2457 w2460] -> w2452
            tunnel: w2451 -> [w2457 w2462]
            tunnel: w2450 -> [_ w2461]
            tunnel: w2449 -> [w2456 w2459]
            tunnel: [w2456 w2458] -> w2448
            frame 0 {
            }
            frame 1, Default {
              n429 = Insert Into Array(array=w2462, index=w2459, new element=w2461) -> (w2460:i32[])
              n430 = Increment(x=w2459) -> (x+1=w2458:i32)
            }
          }
        }
        n431 = local write "Find Array"(w2442) -> ()
        n432 = Empty Array?(array=w2442) -> (empty?=w2441:bool)
        n433 = case shown="True" w2441 {
          tunnel: w2440 -> [_ w2468]
          tunnel: w2442 -> [w2466 _]
          frame False {
            n434 = Index Array(array=w2466, index=0) -> (element=w2464:i32)
            n435 = Bundle By Name(cluster=T2 {"Row"=0, "Column"=0} ("Index Values"), "Row"=w2464) -> (w2463:T2)
            n436 = property on="Table" class="Tbl (strict)"("Index Values"=w2463) -> ()  [unwired: 2 in, 2 out]
          }
          frame True {
            n437 = local read "Table"() -> (w2474:string[][])
            n438 = Index Array(array=w2474, index (col)=4 ("disabled index (col)")) -> (element=w2471:string[])  [unwired: 1 in]
            n439 = for {
              tunnel: w2471 -> [w2483] mode=indexing
              tunnel: w2468 -> [w2482]
              shift-right: [w2480] -> w2469
              shift-left: i32[] [] ("Find Array") -> [w2479]
              shift-right: [w2476] -> _
              shift-left: 0 -> [w2477]
              i -> [w2478]
              n440 = Search and Replace String(input string=w2483, search string=w2482, replace string=w2482) -> (number of replacements=w2481:i32)  [unwired: 5 in, 3 out]
              n441 = case shown="1, Default" w2481 {
                tunnel: [w2485 w2488] -> w2480
                tunnel: w2479 -> [w2485 w2490]
                tunnel: w2478 -> [_ w2489]
                tunnel: w2477 -> [w2484 w2487]
                tunnel: [w2484 w2486] -> w2476
                frame 0 {
                }
                frame 1, Default {
                  n442 = Insert Into Array(array=w2490, index=w2487, new element=w2489) -> (w2488:i32[])
                  n443 = Increment(x=w2487) -> (x+1=w2486:i32)
                }
              }
            }
            n444 = local write "Find Array"(w2469) -> ()
            n445 = Empty Array?(array=w2469) -> (empty?=w2470:bool)
            n446 = case shown="False" w2470 {
              tunnel: w2469 -> [w2493 _]
              frame False {
                n447 = Index Array(array=w2493, index=0) -> (element=w2492:i32)
                n448 = Bundle By Name(cluster=T2 {"Row"=0, "Column"=0} ("Index Values"), "Row"=w2492) -> (w2491:T2)
                n449 = property on="Table" class="Tbl (strict)"("Index Values"=w2491) -> ()  [unwired: 2 in, 2 out]
              }
              frame True {
              }
            }
          }
        }
      }
      event "Next Button": Value Change {
        n450 = event-data() -> ()  [unwired: 1 in, 6 out]
        n451 = local write "Next Button"(FALSE ("Next Button")) -> ()
        n452 = property on="Table" class="Tbl (strict)"() -> ("Index Values"=w2500:T2)  [unwired: 2 in, 2 out]
        n453 = local read "Find Array"() -> (w2497:i32[])
        n454 = Unbundle By Name(w2500) -> ("Row"=w2499:u32)
        n455 = Search 1D Array(1D array=w2497, element=w2499) -> (index of element=w2498:i32)  [unwired: 1 in]
        n456 = case shown="-1" w2498 {
          selector: w2498 -> [_ w2513]
          tunnel: w2497 -> [w2503 w2512]
          frame -1 {
            n457 = Index Array(array=w2503, index=u32 0 ("Row")) -> (element=w2501:i32)
            n458 = Bundle By Name(cluster=T2 {"Row"=0, "Column"=0} ("Index Values"), "Row"=w2501) -> (w2505:T2)
            n459 = property on="Table" class="Tbl (strict)"("Index Values"=w2505) -> ()  [unwired: 2 in, 2 out]
          }
          frame 1, Default {
            n460 = Array Size(array=w2512) -> (size(s)=w2515:i32)
            n461 = Increment(x=w2513) -> (x+1=w2506:i32)
            n462 = Decrement(x=w2515) -> (x-1=w2516:i32)
            n463 = Equal?(x=w2516, y=w2513) -> (x = y?=w2514:bool)
            n464 = Select(t=0 ("f"), s=w2514, f=w2506) -> (s? t:f=w2511:i32)
            n465 = Index Array(array=w2512, index=w2511) -> (element=w2509:i32)
            n466 = Bundle By Name(cluster=T2 {"Row"=0, "Column"=0} ("Index Values"), "Row"=w2509) -> (w2508:T2)
            n467 = property on="Table" class="Tbl (strict)"("Index Values"=w2508) -> ()  [unwired: 2 in, 2 out]
          }
        }
      }
      event "BUTTON_EXIT": Value Change {
        n468 = event-data() -> ()  [unwired: 1 in, 6 out]
      }
    }
  }
